vi "Dashboard Main (1).vi"() -> ()   [LabVIEW 2013]
uses:
  Shoot Profile.ctl
  Autonomous Setpoints.ctl
  Halo Drive.ctl
  Auto Speed Constants.ctl
  Auto Shift Settings.ctl
  Autonomous Center Line Setpoints.ctl
  UDP Dashboard Packet.ctl
  Shoot Location.ctl
  <vilib>/event_ctls.llb/eventvkey.ctl
  <vilib>/Utility/config.llb/Read Key (String).vi
  <vilib>/Utility/config.llb/Read Key (I32).vi
  <vilib>/Utility/config.llb/Write Key (String).vi
  <vilib>/Utility/config.llb/Write Key (I32).vi
  <vilib>/Utility/config.llb/NI_LVConfig.lvlib
  <vilib>/vision/NI_Vision_Development_Module.lvlib
panel:
  in  "Tab Control 2":enum32{"Page 1", "Page 2"}(tab)
  out "Shooter/Output/Vision Mode":bool
  in  "Shooter/Control/Manual RPM":bool=TRUE caption="Manual\n  RPM"
  out "Motor/Output/Elevator Motor":dbl caption="Motor Output"
  in  "Elevator/Manual Elevation":dbl=24.5 caption="Manual"
  in  "Elevator/Feed Angle":dbl=20.0 caption="Feed"
  in  "Elevator/Auto Enabled":bool=TRUE caption="Auto Elevator Enabled"
  out "Shooter/Output/Shooter Ready":bool caption="Shooter Ready"
  in  "Shooter/Pre Feeding":dbl=-0.15 caption="Feed Power"
  in  "Shooter/Main Feeding":dbl=-0.2 caption="Main Feed Pwr"
  in  "Shooter/Control/Manual Main RPM":dbl=4000.0 caption="Target RPM"
  in  "Shooter/Shooter Main":dbl=0.6 caption="Manual Pwr"
  in  "Shooter/Shooter Pre":dbl=0.5 caption="Manual Pwr"
  in  "Shooter/Manual Power":bool caption="Manual Pwr"
  in  "Shooter/Control/Manual Pre RPM":dbl=3500.0 caption="Manual"
  in  "Shooter/Control/RPM Max Percentage":dbl=1.02 caption="RPM Max Percentage"
  in  "Shooter/Control/RPM Min Percentage":dbl=0.99 caption="RPM Min Percentage"
  out "Shooter/Output/Flipper Output":bool caption="Load"
  out "Shooter/Output/RPM Ready":bool caption="RPM"
  out "Elevator/Output/Shoot Angle Ready":bool caption="Elevation"
  in  "Elevator/Manual Elevation Enabled":bool=TRUE caption="Manual\n Angle"
  in  "Elevator/Max Angle":dbl=55.0 caption="Max"
  in  "Elevator/Min Angle":dbl=18.0 caption="Min"
  in  "Elevator/Neutral Angle":dbl=25.8 caption="Neutral Angle"
  out "Shooter/Output/Azimuth Ready":bool caption="Azimuth"
  in  "Azimuth/Auto Enabled":bool caption="Enabled"
  out "Azimuth/Target Delta":dbl caption="Auto Azimuth Delta"
  in  "Azimuth/Tolerance":dbl=3.0 caption="Tolerance"
  out "Azimuth/X Output":dbl caption="X Output"
  out "Elevator/Neutral Angle Ready":bool caption="Ready"
  out "Elevator/Finding Neutral Angle":bool caption="Seeking"
  in  "Elevator/Pyramid Angle":dbl=31.0 caption="Pyramid"
  in  "Elevator/Neutral Enabled":bool=TRUE caption="Neutral\nEnabled"
  out "Shooter/Control/Vision Main RPM":dbl caption="RPM"
  out "Shooter/Control/Vision Pre RPM":dbl caption="Vision"
  out "Elevator/Vision Angle":dbl caption="Vision"
  in  "Shooter/Control/Pyramid Main RPM":dbl=4000.0 caption="Target RPM"
  in  "Shooter/Control/Pyramid Pre RPM":dbl=3500.0 caption="Pyramid"
  in  "Shooter/Control/Full Court Main RPM":dbl=4000.0 caption="Target RPM"
  in  "Shooter/Control/Full Court Pre RPM":dbl=3500.0 caption="Full Court"
  out "Shooter/Output/Pyramid Mode":bool
  out "Shooter/Output/Full Court Mode":bool
  in  "Elevator/Full Court Angle":dbl=25.8 caption="Full Court"
  out "Elevator/Output/Feed Mode":bool
  out "Elevator/Output/Vision Mode":bool
  out "Elevator/Output/Pyramid Mode":bool
  out "Elevator/Output/Full Court Mode":bool
  out "Shooter/Output/Feed Mode":bool
  out "Elevator/Target Angle":dbl caption="Setpoint"
  in  "Camera Settings":T1={"Frate Rate"=30, "Compression"=30, "Size"=1} {"Frate Rate" scale=1.0..30.0; "Size" items=["640x480", "320x240", "160x120"]}
  in  "Dashboard Tab 2":enum32{"Drive", "Debug", "Controls"}(tab)
  out "Elevator Enabled":bool caption="Elevator"
  out "fps":dbl format="%#.1g"
  out "Mbps 2":bool
  in  "DB Camera Config":bool
  in  "Enable":bool=TRUE
  out "Mbps":dbl format="%#.1g"
  out "Camera Image":T2(plugin-control)
  in  "Elevator Angle Offset":dbl(slide)=-0.3 caption="Angle Offset" scale=-5.0..5.0
  out "Azmuth Enabled":bool caption="Azimuth"
  out "Shooter/Output/Shooter Ready 2":bool caption="Shooter Ready"
  out "Shooter/Output/Flipper Output 2":bool caption="Load"
  out "Shooter/Output/RPM Ready 2":bool caption="RPM"
  out "Elevator/Output/Shoot Angle Ready 2":bool caption="Elevation"
  out "Shooter/Output/Azimuth Ready 2":bool caption="Azimuth"
  out "Elevator/Output/Target Angle 2":dbl caption="Target"
  out "Elevator/Angle 2":dbl caption="Angle"
  out "Vision/Target Found":bool caption="Target\nFound"
  out "Shoot Distance":dbl
  out "Gyro Angle":dbl(knob) caption="Gyro" scale=0.0..360.0
  out "Drive Gear":dbl caption="Gear"
  out "Auto/Load Ramp Down":bool caption="Ramp Down"
  in  "Dashboard Tab":T3(tab)
  out "Encoder/Right Ticks":dbl caption="Right"
  out "Encoder/Left Ticks":dbl caption="Left"
  out "Encoder/Right Speed":dbl caption="Right"
  out "Encoder/Left Speed":dbl caption="Left"
  out "Auto/Shooter Mode":string="--------" caption="Shooter Mode"
  out "Drive/Gear":dbl caption="Gear"
  out "Encoder/Right Dist":dbl caption="Right"
  out "Encoder/Left Dist":dbl caption="Left"
  out "Encoder/Average Dist":dbl caption="Encoder Distance"
  out "Sensor/Disc Count":dbl caption="Discs" format="%#_1f"
  out "Sensor/Gyro/Angle":dbl(knob) caption="Gyro" scale=0.0..360.0
  out "Auto/Disc Mode":string="--------" caption="Disc Mode"
  out "Lift/Ratchet Locked":bool caption="Ratchet Locked"
  out "Shoot Active Vision":bool caption="Ratchet Locked"
  out "Shoot Active Pyramid":bool caption="Ratchet Locked"
  out "Shoot Active Full Court":bool caption="Ratchet Locked"
  out "Shoot Active Half Court":bool caption="Ratchet Locked"
  out "Shoot Active Back Corner":bool caption="Ratchet Locked"
  out "Shoot Active Front Corner":bool caption="Ratchet Locked"
  in  "Shoot Pyramid":T4={"Pre RPM"=2800.0, "Main RPM"=3300.0, "Angle"=28.0} caption="Pyramid"
  in  "Shoot Full Court":T4={"Pre RPM"=4500.0, "Main RPM"=4800.0, "Angle"=12.0} caption="Full Court"
  in  "Shoot Half Court":T4={"Pre RPM"=3600.0, "Main RPM"=4100.0, "Angle"=16.4} caption="Half Court"
  in  "Shoot Front Corner":T4={"Pre RPM"=3600.0, "Main RPM"=4100.0, "Angle"=19.900000000000002} caption="Front Corner"
  in  "Shoot Front":T4={"Pre RPM"=3600.0, "Main RPM"=4100.0, "Angle"=23.5} caption="Front"
  out "Sensor/Shooter Pot/Value":dbl caption="Pot Voltage"
  in  "Angle Equation x0":dbl=51.125
  in  "Angle Equation x1":dbl=-2.486
  in  "Angle Equation x2":dbl=0.0385 caption="Vision Angle Equation"
  in  "Manual Elevation Enabled":bool=TRUE
  in  "Manual Angle":dbl=16.4
  out "Vision Elevation":dbl caption="Vision Angle"
  in  "Feed Angle":dbl=20.0
  in  "Neutral Angle":dbl=16.4
  in  "Shoot Vision":T4={"Pre RPM"=3600.0, "Main RPM"=4100.0, "Angle"=16.4}
  in  "Shooter/Control/Manual Dist Enabled":bool caption="Manual Distance"
  in  "Shooter/Control/Manual Dist":dbl=12.0 caption="Manual Distance"
  out "Camera Distance 2":dbl caption="Camera Dist"
  out "Shoot Distance 2":dbl caption="Shoot Dist"
  out "Shooter/Control/Target Pre RPM":dbl caption="Setpoint"
  out "Shooter/Control/Target Main RPM":dbl caption="RPM"
  out "Shooter/Output/Pre RPM":dbl caption="Sensor"
  out "Shooter/Output/Pre":dbl caption="Output"
  out "Shooter/Output/Main":dbl caption="Motor\nOutput"
  out "Shooter/Output/Main RPM":dbl caption="RPM"
  out "Elevator/Angle 3":dbl caption="Angle"
  out "Elevator/Output/Target Angle 3":dbl caption="Target"
  out "Shoot Active Front":bool caption="Ratchet Locked"
  in  "Shoot Back Corner":T4={"Pre RPM"=3600.0, "Main RPM"=4100.0, "Angle"=13.300000000000006} caption="Back Corner"
  in  "Angle Tolerance":dbl=0.1
  in  "Unjam Servo Angle":dbl=60.0
  in  "Potentiometer Angle":cluster{"Pot M":dbl, "Pot B":dbl}={"Pot M"=42.09, "Pot B"=-65.397}
  out "Elevator/Output/Target Angle":dbl caption="Target"
  in  "Sensor/Shooter Pot/Value":dbl caption="Shooter Pot"
  out "Elevator/Angle":dbl caption="Angle"
  in  "Halo Drive":T5={"Gains"={"Quickturn_Sens_Low"=1.2, "Quickturn_Sens_High"=0.85, "Speedturn_Sens_Low"=1.5, "Speedturn_Sens_High"=2.0}, "QuickTurn Const"=0.25, "Loading Throttle Limit"=0.5}
  in  "Toggle Ears Delay":dbl=-1.0
  in  "Left Roller Pwr":dbl=0.9
  in  "Right Roller Pwr":dbl=0.8
  in  "Toggle Ears Distance":dbl=2.0
  in  "Auto Shift":T6={"Enabled"=FALSE, "Upshift Speed"=6.0, "Downshift Speed"=2.0, "Upshift Throttle"=0.6000000000000001, "Turn Power Diff"=0.7, "Motor Limit"=100.0, "Encoder Limit"=1500.0}
  in  "Shooting Delays":T7={"Unjam On"=200.0, "Unjam Off"=200.0, "Flipper On"=200.0, "Flipper Off"=0.0, "Hopper Up"=300.0}
  in  "Auto Reverse Speed":dbl=0.5
  in  "Autonomous Setpoints":T8={"Shoot Angle 1"=14.8, "Initial Delay"=0.0, "Disc Count 1"=3.0, "Shoot Time 1"=8000.0, "Distance 1"=6.5, "Two Disc Distance 1"=4.0, "Distance 2"=12.5, "Two Disc Distance 2"=6.0, "Distance 3"=-11.8, "Two Disc Distance 3"=0.0, "Shoot Angle 3"=22.5, "Disc Count 3"=5.0, "Shoot Time 3"=15000.0, "Distance 4"=0.0, "Two Disc Distance 4"=0.0, "Low Gear"=TRUE, "Shoot 1 Post Delay"=250.0}
  in  "Auto Speed Constants":T9={"Slowing Distance"=0.5, "High Speed"=0.8999999999999999, "Rampup Time"=500.0, "Low Speed"=0.5, "High Speed (Reverse)"=0.8999999999999999}
  in  "Auto Stop Throttle":dbl
  in  "Auto Stop Duration (ms)":dbl
  in  "Auto-Center Line":T10={"Arc Turn x-axis"=0.0, "Arc Turn y-axis"=0.8999999999999999, "Arc Turn Distance"=-11.0, "Distance 1"=11.0, "Two Disc Distance 1"=0.0, "Distance 2"=-2.0, "Two Disc Distance 2"=0.0, "Spin Angle"=-70.0, "Spin Angle tolerance"=5.0, "Spin y-axis"=0.0, "Spin Distance"=0.0, "Center Line Enabled"=FALSE, "Distance 3"=11.999999999999998, "Two Disc Distance 3"=0.0, "Spin Angle 2"=85.0, "Spin Angle tolerance 2"=15.0, "Spin y-axis 2"=0.0, "Spin Distance 2"=0.0, "Shoot Angle 1"=14.6, "Disc Count 1"=3.0, "Shoot Time 1"=8000.0, "Shoot Angle 3"=18.4, "Disc Count 3"=5.0, "Shoot Time 3"=15000.0, "Low Gear"=TRUE}
  in  "Slider":dbl(slide) scale=0.0..100.0 scale format="%#_3g"
  in  "On/Off":bool caption="Solenoid"
  in  "Test Name":u16(ring) items=["Select the test to run...", "Example Test", "-------------------------------", "List of tests is built in robot code.", "Replace with your own automated tests."]
  in  "Test Tree":string(tree)
  in  "Motor":cluster{"Value":dbl, "Enable":bool} {"Value" scale=-1.0..1.0 scale format="%#_3g"}
  out "Progress":T11 {"Test Progress" scale=0.0..100.0}
  in  "Rev/Fwd":cluster{"Forward":bool, "Reverse":bool}
  in  "Ring":u16(ring) items=["Auto", "Fixed indoor", "Fixed outdoor 1", "Fixed outdoor 2", "Fixed fluorescent 1", "Fixed fluorescent 2", "Hold current"]
  in  "Listbox":i32(listbox)
  out "Tree":string(tree)
  out "UDP packet length":i32
  in  "Auton Distance output range\nCenter Line":cluster{"output high":dbl, "output low":dbl}={"output high"=1.0, "output low"=-1.0}
  in  "Auton Distance PID gains\nHigh Gear":T12={"proportional gain (Kc)"=0.26, "integral time (Ti, min)"=0.018000000000000002, "derivative time (Td, min)"=0.0}
  in  "Elevator PID Gains":T12={"proportional gain (Kc)"=0.2, "integral time (Ti, min)"=0.0, "derivative time (Td, min)"=0.002}
  in  "Elevator PID Output Range":cluster{"output high":dbl, "output low":dbl}={"output high"=1.0, "output low"=-1.0}
  in  "Auton Steer PID gains":T12={"proportional gain (Kc)"=0.4, "integral time (Ti, min)"=0.0, "derivative time (Td, min)"=0.002}
  in  "Auton Steer output range":cluster{"output high":dbl, "output low":dbl}={"output high"=0.5, "output low"=-0.5}
  in  "Auton Spin output range":cluster{"output high":dbl, "output low":dbl}={"output high"=1.0, "output low"=-1.0}
  in  "Auton Spin PID gains":T12={"proportional gain (Kc)"=0.4, "integral time (Ti, min)"=0.0, "derivative time (Td, min)"=0.0}
  in  "Auton Distance PID gains\nLow Gear":T12={"proportional gain (Kc)"=0.9999999999999999, "integral time (Ti, min)"=0.007, "derivative time (Td, min)"=0.0}
  in  "Auton Distance output range":cluster{"output high":dbl, "output low":dbl}={"output high"=0.93, "output low"=-0.93}
  in  "Auton Distance Threshold":dbl=0.5
  in  "Auton Velocity Cutoff":dbl=2.0
  in  "Mask":bool
  out "Image Display":T2(plugin-control)
  in  "View":bool
  in  "Tab Control":enum32{"Variables", "Calibration"}(tab)
  out "Target Info":T13(array[cluster])
  in  "Particle Count Limit":i32=8
  in  "Area Size Limit %":dbl=0.5
  in  "Score Limits":T14={"Rect Coverage"=60.0, "X Edge Strength"=40.0, "Y Edge Strength"=60.0, "Center"=75.0, "Outer"=75.0}
  in  "Camera Type":enum16{"206", "1011"}(ring)=enum."1011"
  out "Center Position":cluster{"X":dbl, "Y":dbl}
  out "Vision Distance (ft)":dbl caption="Distance (ft)"
  out "Center":bool
  out "Position X":dbl
  in  "Default Distance (ft)":dbl=14.0
  in  "Position to\nGyro constant":dbl=21.75
  in  "Azimuth Offset":dbl
  out "Azimuth/Target Delta 2":dbl caption="Auto Azimuth Delta"
  out "Azimuth/X Output 2":dbl caption="X Output"
  in  "Image Filter Values":T15={"Hue"=105, "Saturation"=255, "Luminance"=235, "Margins"={"Hue"=80, "Val"=80, "Sat"=0}} {"Margins"."Sat" scale=0.0..80.0; "Margins"."Val" scale=0.0..80.0; "Margins"."Hue" scale=0.0..80.0; "Hue" scale=0.0..255.0}
  out "Image Filter Ranges":T16
  out "Battery Value":dbl(slide) scale=0.0..14.0 scale format="%#_2e"
  out "Battery":sgl(graph)
  out "JS1 Z":dbl(slide) scale=-1.0..1.0 scale format="%#_2e"
  out "JS2 Z":dbl(slide) scale=-1.0..1.0 scale format="%#_2e"
  out "Joystick 1":cluster{"X":dbl, "Y":dbl}[](graph)
  out "Joystick 2":cluster{"X":dbl, "Y":dbl}[](graph)
  out "JS Buttons 1":T17
  out "JS Buttons 2":T17
  out "MotorSlide4":dbl(slide) scale=-1.0..1.0 scale format="%#_2e"
  out "MotorSlide3":dbl(slide) scale=-1.0..1.0 scale format="%#_2e"
  out "MotorSlide2":dbl(slide) scale=-1.0..1.0 scale format="%#_2e"
  in  "MotorName3":string="Front Left"
  in  "MotorName4":string="Front Right"
  in  "MotorName1":string="Rear Left"
  in  "MotorName2":string="Rear Right"
  out "MotorChart4":dbl(graph)
  out "MotorChart3":dbl(graph)
  out "MotorChart2":dbl(graph)
  out "MotorSlide1":dbl(slide) scale=-1.0..1.0 scale format="%#_2e"
  out "MotorChart1":dbl(graph)
  out "Robot IP":string
  out "Mode":T18(ring)=enum."Auto Disabled"
  out "Camera IP":string
  in  "Viewer":T19(tab)
  out "Image Error Message":string="Timeout in Camera Communications"
  out "Buttons 1":cluster{"1":bool, "2":bool, "3":bool}
  out "Kinect 1":cluster{"X":dbl, "Y":dbl, "Z":dbl} {"X" scale=1.0..-1.0; "Y" scale=1.0..-1.0; "Z" scale=1.0..-1.0}
  out "Buttons 2":cluster{"1":bool, "2":bool, "3":bool}
  out "Kinect 2":cluster{"X":dbl, "Y":dbl, "Z":dbl} {"X" scale=1.0..-1.0; "Y" scale=1.0..-1.0; "Z" scale=1.0..-1.0}
  out "Version":string
  out "Skeleton Picture":picture
  out "Players":i8
  # "Pre"
  # "Main"
  # "Neutral"
  # "Vision: 3500, 4000\nPyramid: 2800, 3200  39.1\nFull Court: 4300, 4800 18"
  # "Shooter"
  # "Elevator"
  # "Distance"
  # "Ticks"
  # "Speed"
  # "RPM"
  # "NOTE: used as\nBack angle"
  # "Pre RPM"
  # "Main RPM"
  # "Angle"
  # "Dpad UP"
  # "Elevator UP"
  # "Elevator DOWN"
  # "Dpad LEFT"
  # "Dpad RIGHT"
  # "[DISABLED]"
  # "Elevator"
  # "Whiteboard:                               y = -2.6332x + 68.073\nTesting 2.23.13                           y = 0.2002x2 - 7.6337x + 101.11\nTesting 2.24.13                           y = 0.2086x2 - 7.5585x + 94.621\nField Test (Orch room) 3.2.13  y = 0.0733x2 - 3.2492x + 59.29\nField Test (Orch room) 3.3.13  y = 0.0782x2 - 3.7527x + 65.268\nLonestar Thursday 3.7.13         y = 0.0872x2 - 3.5994x + 63.288 \nLonestar Friday 3.8.13               y = 0.178x2 - 6.8038x + 91.639\nPrePeachtree 3.11.13                 y = -0.0522x2 + 0.9287x + 27.34 \nPeachtree Thurs 3.14.13           y = -0.0766x2 + 0.7339x + 30.218\nPeachtree Thurs 3.14.13 PM    y = 0.0385x2 - 2.486x + 51.125"
  # "Dpad DOWN"
  # "x^2"
  # "x"
  # "Start angle: 28"
  # "Duration to move Lift Piston up\nat beginning of teleop (-1 to disable)"
  # "Quickturn - LOW throttle"
  # "Speedturn - HIGH throttle"
  # "Volts -> Degrees\ny = Mx + B"
  # "throttle value where Speedturn activates"
  # "Max throttle value when ramp is down"
  # "2 Corner:\nDistance 1 = 18\nDistance 2 = 0\nSpin 2 = 105\nDistance 3 = 10"
  # "Distance before stopping,\nswitch to low speed"
  # "Time to get to full speed (ms)"
  # "7.13.13\nP=0.6\nI =0.006\nD=0"
  # "2.23.13\nP=0.068\nI =0.8\nD=0.008\nTolerance=3deg"
  # "Original values:\np=0.3, range [-1, 1]"
  # "Original values:\n1.2, 1\n1.5, 1.7"
  # "Driver  [USB 1]"
  # "Manipulator [USB 2]"
  # "Drive & Motors"
  # "Simple Shoot: [2] (uses back pyramid angle)\nAdvanced Shoot:\n     Back of Pyramid:  [D-Pad Down] + [2]\n     Front of Pyramid: [D-Pad Up] + [2]\n     Front Corner: [11 Up] + [2]\n     Back Corner: [11 Down] + [2]\n     Half Court: [D-Pad Left] + [2]\n     Full Court:  [D-Pad Right] + [2]\nNOTE: [2] activates flipper (other button\nwarms up shooter & angle)\n\nLeft Roller -    [5] Forward; [7] Backward\nRight Roller - [6] Forward; [8] Backward\n\nFront Feeding - [3]\n\nManual Flipper - [9]\nManual Hopper - [1]\nManual Unjam - [12 Down]\nManual Elevator - [10] + [11 Up/Down]\n^(disables auto elevator, push [11] to re-enable)\nEnable Auto Elevator - [Push 11]\n\nVision Enabled - [4]*  (disabled by default)\n*toggle button"
  # "Drive:\n     Throttle - [11 Up/Down]\n     Steering - [12 Left/Right]\n     Gear Shift - [5]*\n     (starts in High gear)\n\n10pt Lift Piston - [7]* or [2]*\n\nAuto Load - [6]\nLoad Ramp Down - [8]\n\n*toggle button"
  # "Note: Most commonly used controls are listed first"
  # "Robot IP:"
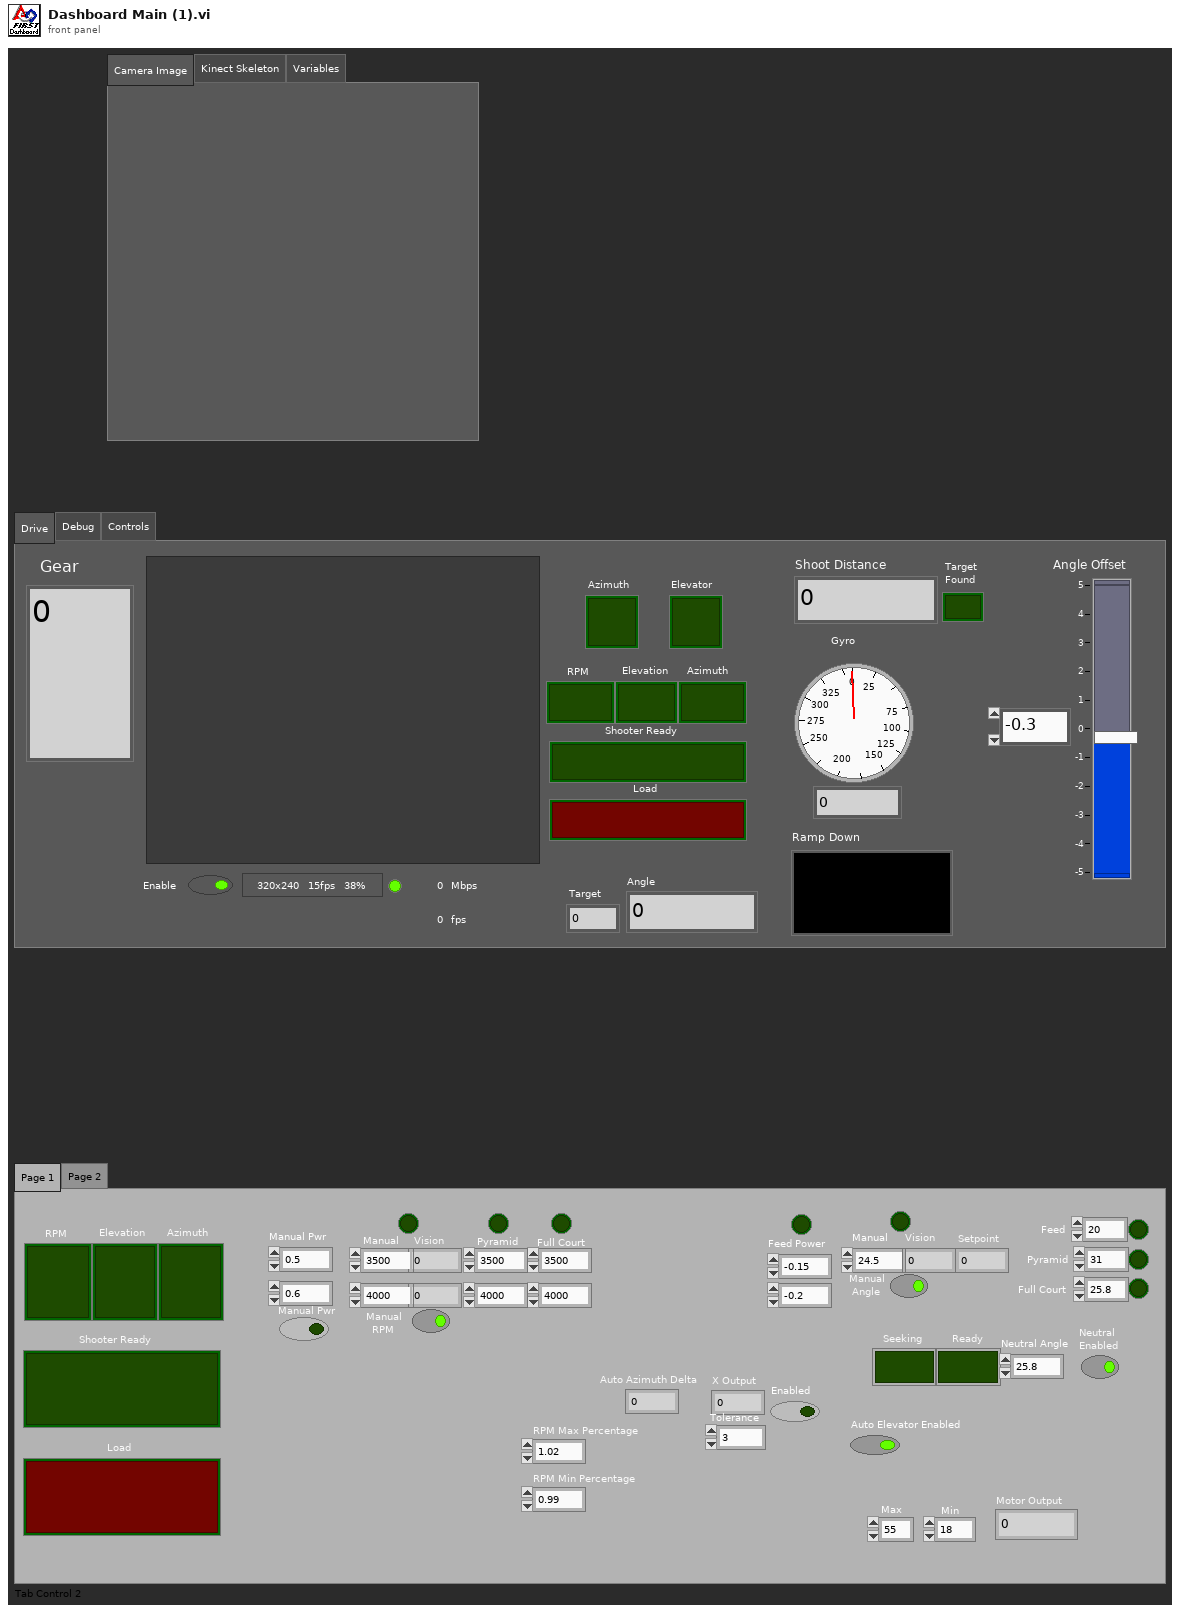
[diagram p1: front panel]
types:
  T1 = cluster{"Frate Rate":i32, "Compression":i32, "Size":u16}
  T2 = typedef "IMAQ Image.ctl" = refnum<image>
  T3 = enum32{"Operation", "Shooter", "Auto", "Autonomous", "Test", "Variables", "PID", "Vision"}
  T4 = typedef "Shoot Profile.ctl" = cluster{"Pre RPM":dbl, "Main RPM":dbl, "Angle":dbl}
  T5 = typedef "Halo Drive.ctl" = cluster{"Gains":cluster{"Quickturn_Sens_Low":dbl, "Quickturn_Sens_High":dbl, "Speedturn_Sens_Low":dbl, "Speedturn_Sens_High":dbl}, "QuickTurn Const":dbl, "Loading Throttle Limit":dbl}
  T6 = typedef "Auto Shift Settings.ctl" = cluster{"Enabled":bool, "Upshift Speed":dbl, "Downshift Speed":dbl, "Upshift Throttle":dbl, "Turn Power Diff":dbl, "Motor Limit":dbl, "Encoder Limit":dbl}
  T7 = cluster{"Unjam On":dbl, "Unjam Off":dbl, "Flipper On":dbl, "Flipper Off":dbl, "Hopper Up":dbl}
  T8 = typedef "Autonomous Setpoints.ctl" = cluster{"Shoot Angle 1":dbl, "Initial Delay":dbl, "Disc Count 1":dbl, "Shoot Time 1":dbl, "Distance 1":dbl, "Two Disc Distance 1":dbl, "Distance 2":dbl, "Two Disc Distance 2":dbl, "Distance 3":dbl, "Two Disc Distance 3":dbl, "Shoot Angle 3":dbl, "Disc Count 3":dbl, "Shoot Time 3":dbl, "Distance 4":dbl, "Two Disc Distance 4":dbl, "Low Gear":bool, "Shoot 1 Post Delay":dbl}
  T9 = typedef "Auto Speed Constants.ctl" = cluster{"Slowing Distance":dbl, "High Speed":dbl, "Rampup Time":dbl, "Low Speed":dbl, "High Speed (Reverse)":dbl}
  T10 = typedef "Autonomous Center Line Setpoints.ctl" = cluster{"Arc Turn x-axis":dbl, "Arc Turn y-axis":dbl, "Arc Turn Distance":dbl, "Distance 1":dbl, "Two Disc Distance 1":dbl, "Distance 2":dbl, "Two Disc Distance 2":dbl, "Spin Angle":dbl, "Spin Angle tolerance":dbl, "Spin y-axis":dbl, "Spin Distance":dbl, "Center Line Enabled":bool, "Distance 3":dbl, "Two Disc Distance 3":dbl, "Spin Angle 2":dbl, "Spin Angle tolerance 2":dbl, "Spin y-axis 2":dbl, "Spin Distance 2":dbl, "Shoot Angle 1":dbl, "Disc Count 1":dbl, "Shoot Time 1":dbl, "Shoot Angle 3":dbl, "Disc Count 3":dbl, "Shoot Time 3":dbl, "Low Gear":bool}
  T11 = cluster{"Test Progress":u8, "Test Progress Text":string}
  T12 = cluster{"proportional gain (Kc)":dbl, "integral time (Ti, min)":dbl, "derivative time (Td, min)":dbl}
  T13 = cluster{"Center Position":cluster{"X":dbl, "Y":dbl}, "Distance (ft)":dbl, "Center":bool}[]
  T14 = cluster{"Rect Coverage":dbl, "X Edge Strength":dbl, "Y Edge Strength":dbl, "Center":dbl, "Outer":dbl}
  T15 = cluster{"Hue":i32, "Saturation":i32, "Luminance":i32, "Margins":cluster{"Hue":i32, "Val":i32, "Sat":i32}}
  T16 = cluster{"Hue":cluster{i32, i32}, "Sat":cluster{i32, i32}, "Lum":cluster{i32, i32}}
  T17 = cluster{bool, bool, bool, bool, bool, bool, bool, bool, bool, bool, bool, bool}
  T18 = enum8{"Tele-Op Disabled", "Tele-Op Enabled", "Auto Disabled", "Auto Enabled", "Test Disabled", "Test Enabled", ""}
  T19 = enum32{"Camera Image", "Kinect Skeleton", "Variables"}
  T20 = typedef "UDP Dashboard Packet.ctl" = cluster{"Feed Angle":dbl, "Neutral Angle":dbl, "Autonomous Setpoints":T8, "Auto Shift":T6, "Elevator Angle Offset":dbl, "Potentiometer Angle":cluster{"Pot M":dbl, "Pot B":dbl}, "Shoot Setpoints":cluster{"Vision":T4, "Back Corner":T4, "Front":T4, "Front Corner":T4, "Half Court":T4, "Full Court":T4, "Pyramid":T4}, "Halo Drive":T5, "Auto Speed Constants":T9, "Shooting Delays":cluster{"Unjam On":dbl, "Unjam Off":dbl, "Flipper On":dbl, "Flipper Off":dbl, "Hopper Up":dbl}, "Left Roller Pwr":dbl, "Right Roller Pwr":dbl, "Elevator PID Gains":cluster{"proportional gain (Kc)":dbl, "integral time (Ti, min)":dbl, "derivative time (Td, min)":dbl}, "Elevator PID Output Range":cluster{"output high":dbl, "output low":dbl}, "Elevator Angle Tolerance":dbl, "Toggle Ears Delay":dbl, "Toggle Ears Distance":dbl, "Unjam Servo Angle":dbl, "Auton Steer PID gains":cluster{"proportional gain (Kc)":dbl, "integral time (Ti, min)":dbl, "derivative time (Td, min)":dbl}, "Auton Steer output range":cluster{"output high":dbl, "output low":dbl}, "Auto Reverse Speed":dbl, "Auto Stop Throttle":dbl, "Auto Stop Duration":dbl, "Spin output range":cluster{"output high":dbl, "output low":dbl}, "Spin PID gains":cluster{"proportional gain (Kc)":dbl, "integral time (Ti, min)":dbl, "derivative time (Td, min)":dbl}, "Auto-Center Line":T10, "Auton Distance PID gains Low Gear":cluster{"proportional gain (Kc)":dbl, "integral time (Ti, min)":dbl, "derivative time (Td, min)":dbl}, "Auton Distance output range":cluster{"output high":dbl, "output low":dbl}, "Auton Distance Threshold":dbl, "Auton Velocity Cutoff":dbl, "Auton Distance output range Center Line":cluster{"output high":dbl, "output low":dbl}, "Auton Distance PID gains High Gear":cluster{"proportional gain (Kc)":dbl, "integral time (Ti, min)":dbl, "derivative time (Td, min)":dbl}}
  T21 = typedef "Image Type" = u32
  T22 = enum32{"Operation", "Test", "Checklist", "Shooter", "Elevator", "Motors", "Solenoids", "Auto"}
  T23 = enum32{"Operation", "Test", "Checklist", "Shooter", "Motors"}
  T24 = typedef "LVBoundsTypeDef.ctl" = cluster{"Width":u32, "Height":u32}
  T25 = typedef "SkeletonTrackState.ctl" = enum32{"NotTracked", "PositionOnly", "Tracked"}
  T26 = cluster{"TrackingState":u8[], "Position":cluster{"x":sgl, "y":sgl, "z":sgl}, cluster{"x":sgl, "y":sgl, "z":sgl, sgl}[], "TrackState":T25}
  T27 = cluster{cluster{"ScaledToPercentRange":dbl, "ScaledToPercentRange":dbl, "ScaledToPercentRange":dbl}, cluster{bool, bool, bool}}[]
  T28 = cluster{cluster{"ScaledToPercentRange":dbl, "ScaledToPercentRange":dbl, "ScaledToPercentRange":dbl}, cluster{bool, bool, bool}}
  T29 = cluster{"ScaledToPercentRange":dbl, "ScaledToPercentRange":dbl, "ScaledToPercentRange":dbl}
  T30 = typedef "LVRectTypeDef.ctl" = cluster{"Left":i16, "Top":i16, "Right":i16, "Bottom":i16}
  T31 = cluster{"Center Position":cluster{"X":dbl, "Y":dbl}, "Distance (ft)":dbl, "Center":bool}
  T32 = cluster{"Competition mode":bool, "Robot Link":bool, "Autonomous":bool, "Enabled":bool, "E-Stop":bool, "Simulated":bool, "TestMode":bool, "Docked Window":bool}
  T33 = cluster{"Boolean Array[0]":bool, "Boolean Array[1]":bool, "Boolean Array[2]":bool, "Boolean Array[3]":bool, "Boolean Array[4]":bool, "Boolean Array[5]":bool, "Boolean Array[6]":bool, "Boolean Array[7]":bool, "Boolean Array[8]":bool, "Boolean Array[9]":bool, "Boolean Array[10]":bool, "Boolean Array[11]":bool}
  T34 = typedef "NI_LVConfig.lvlib/Config Data RefNum.ctl" = refnum<k1>
  T35 = typedef "eventvkey.ctl" = enum16{"ASCII", "Enter", "Return", "Shift", "Ctrl", "Alt", "Cmd", "Opt", "Caps", "NumLock", "Clear", "Break", "Up", "Down", "Left", "Right", "Insert", "Delete", "Home", "End", "PageUp", "PageDown", "Escape", "Help", "Pause", "ScrollLock", "F1", "F2", "F3", "F4", "F5", "F6", "F7", "F8", "F9", "F10", "F11", "F12", "F13", "F14", "F15", "F16", "F17", "F18", "F19", "F20", "F21", "F22", "F23", "F24", "Play", "VolumeUp", "VolumeDown", "Mute", "Two Byte Char"}
  T36 = typedef "Shoot Location.ctl" = enum16{"Vision", "Front", "Front Corner", "Back Corner", "Half Court", "Full Court", "Pyramid"}
  T37 = cluster{"Vision":T4, "Back Corner":T4, "Front":T4, "Front Corner":T4, "Half Court":T4, "Full Court":T4, "Pyramid":T4}
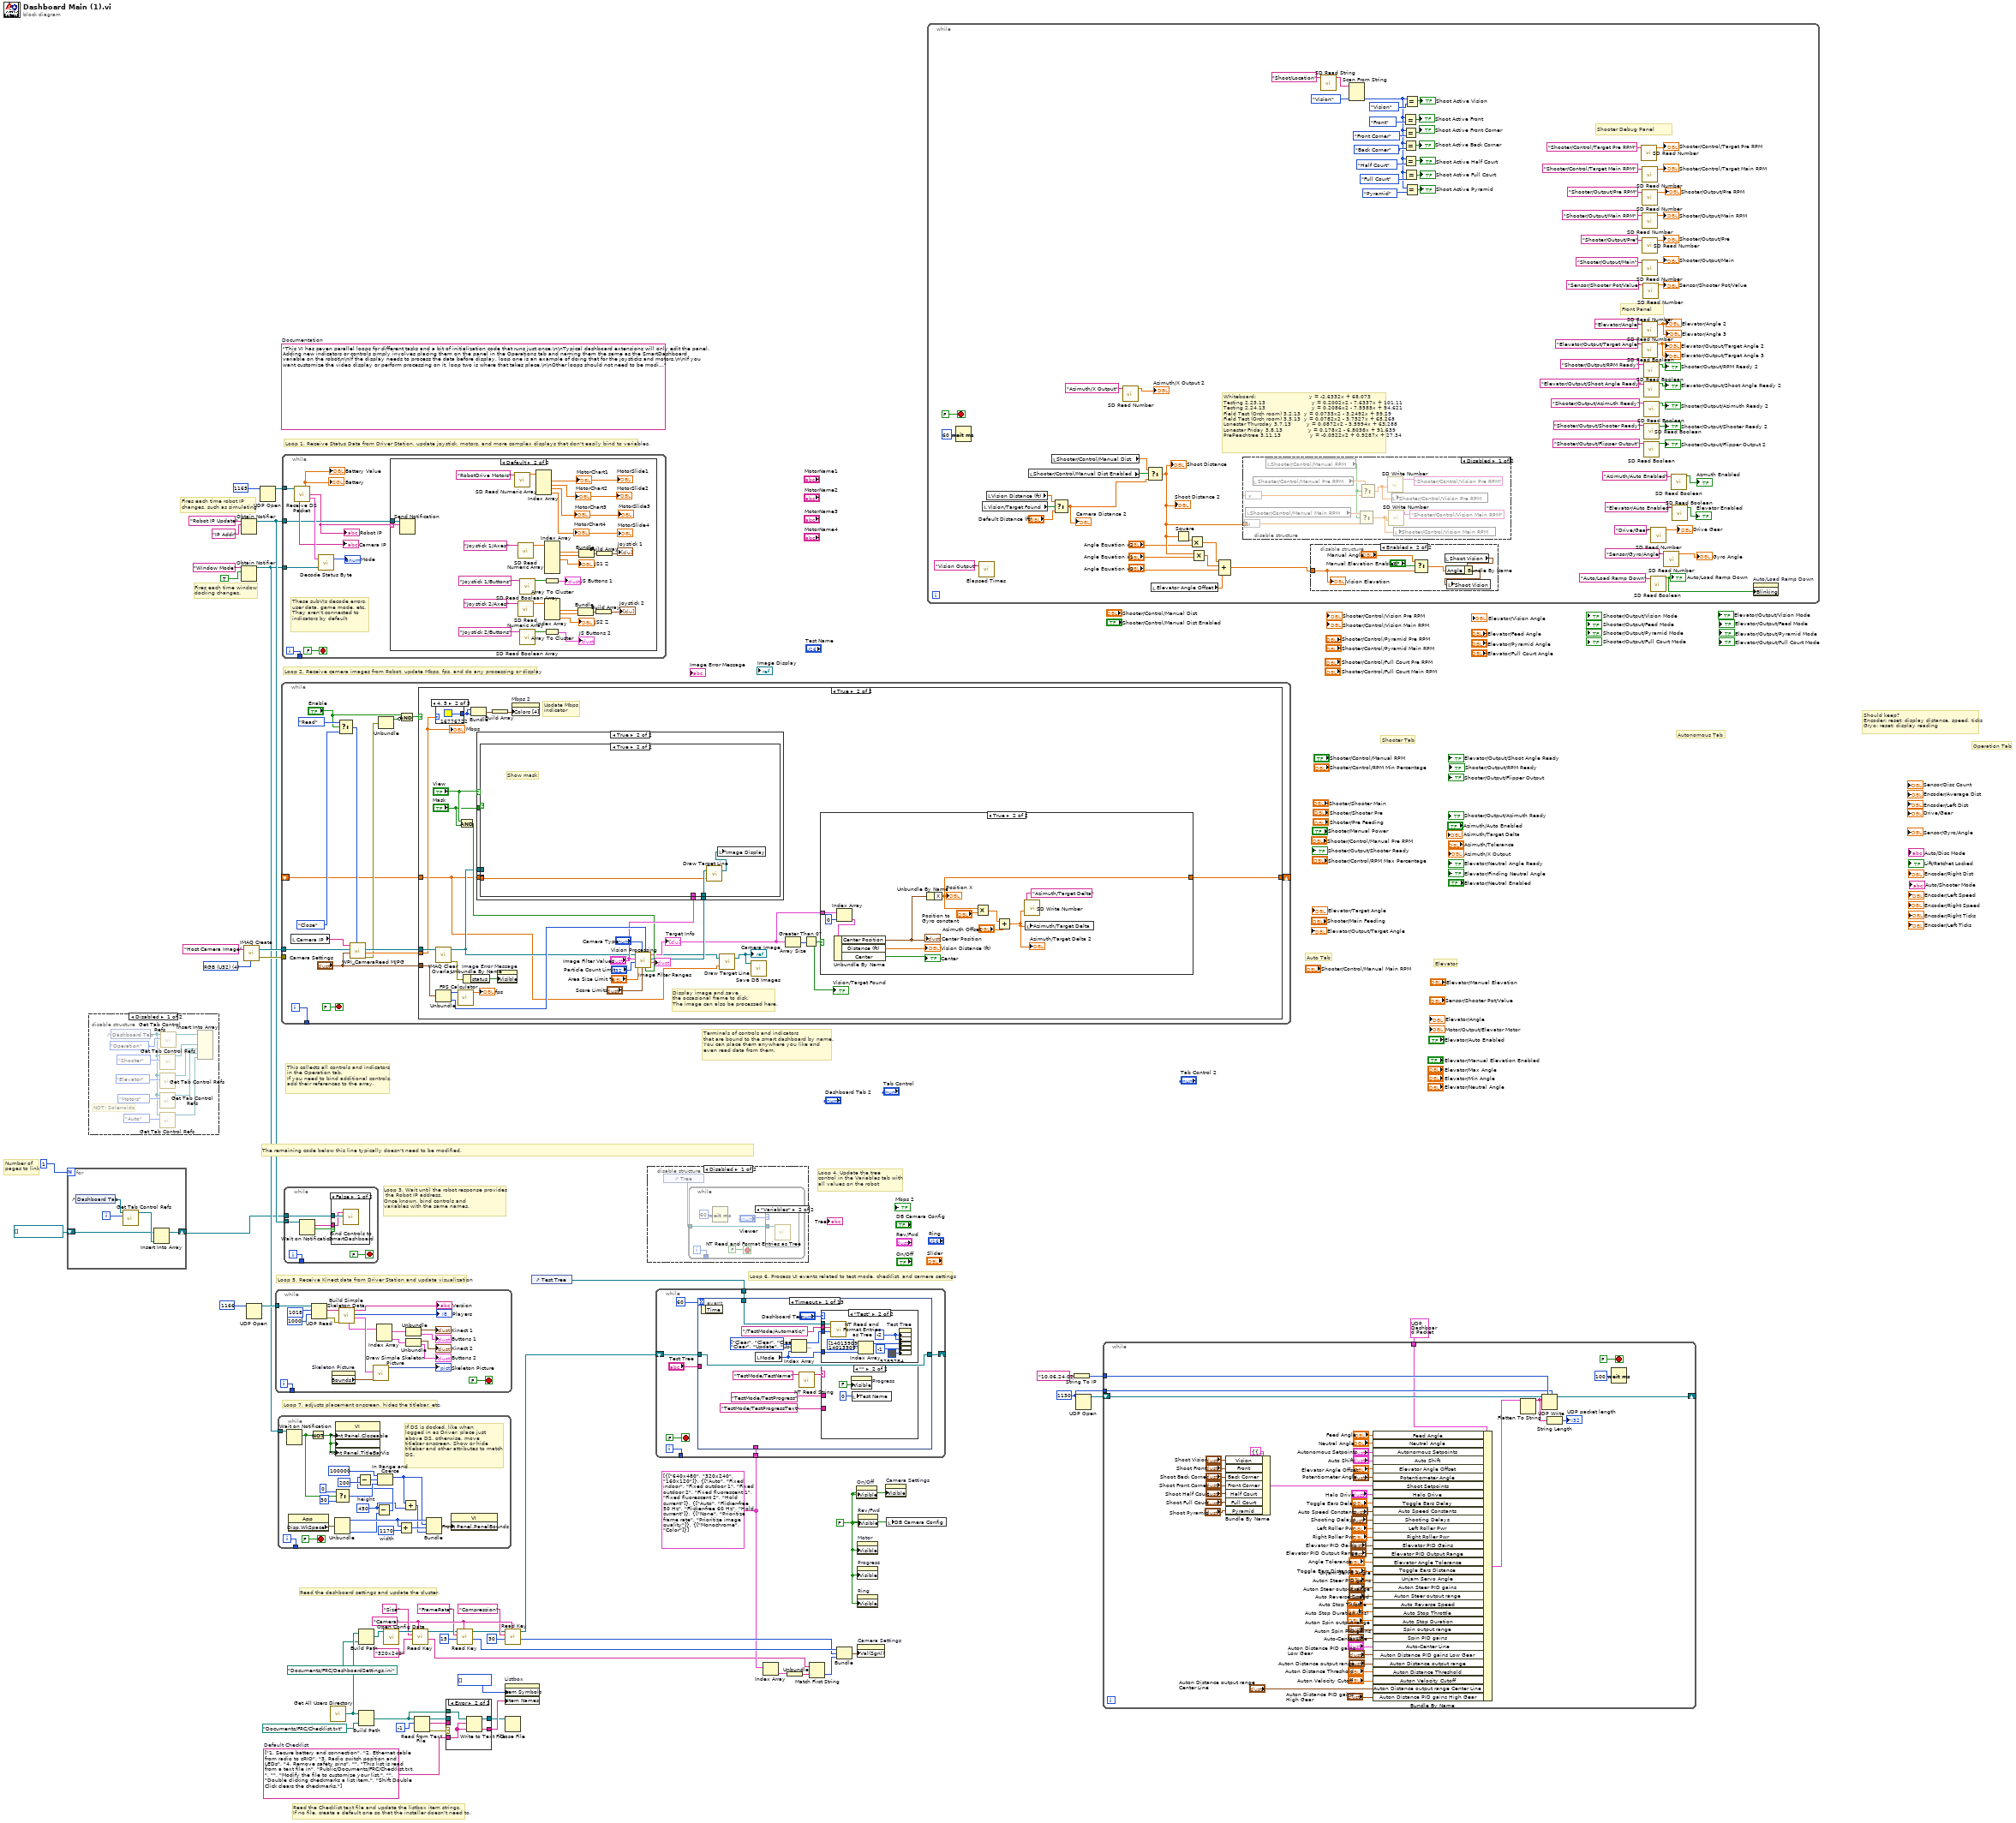
[diagram p0: block diagram]
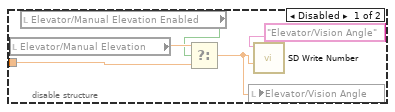
[diagram p2: hidden frame]
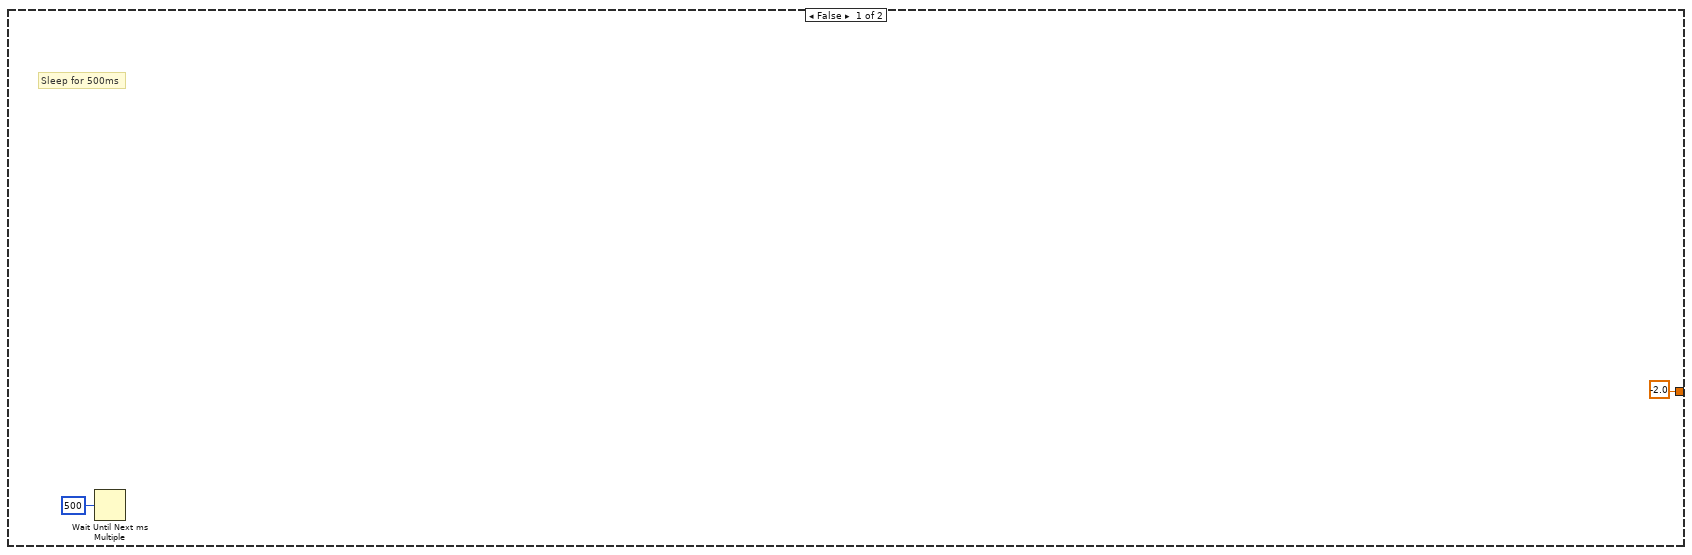
[diagram p8: hidden frame]
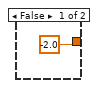
[diagram p9: hidden frame]
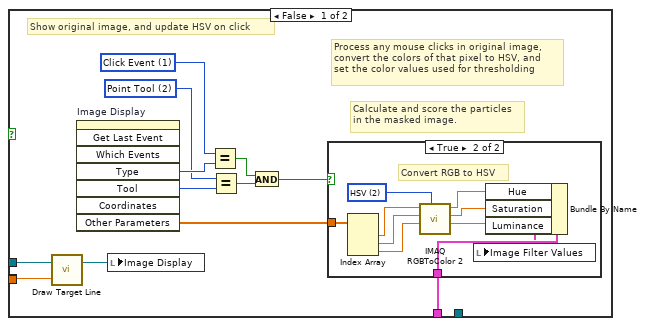
[diagram p11: hidden frame]
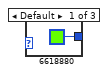
[diagram p13: hidden frame]
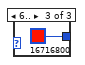
[diagram p14: hidden frame]
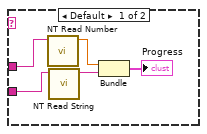
[diagram p17: hidden frame]
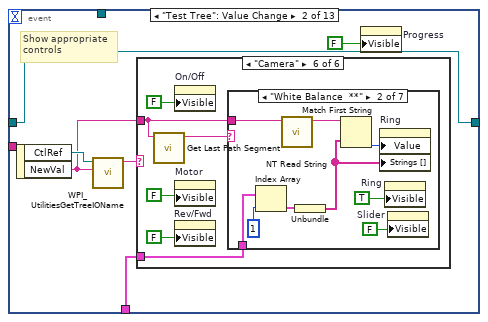
[diagram p18: hidden frame]
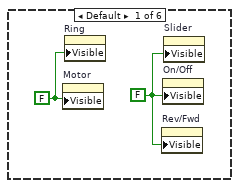
[diagram p19: hidden frame]
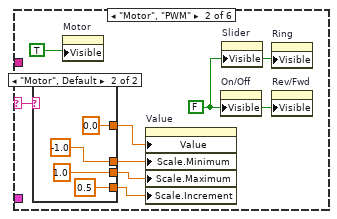
[diagram p20: hidden frame]
diagram:
  w2 = u16 1130 ("port")
  w28 = "Camera"
  w20 = cluster{string[]}[] [{["640x480", "320x240", "160x120"]}, {["Auto", "Fixed indoor", "Fixed outdoor 1", "Fixed outdoor 2", "Fixed fluorescent 1", "Fixed fluorescent 2", "Hold current"]}, {["Auto", "Flicker-free 50 Hz", "Flicker-free 60 Hz", "Hold current"]}, {["None", "Prioritize frame rate", "Prioritize image quality"]}, {["Monochrome", "Color"]}]
  w36 = string[] ["1. Secure battery and connection", "2. Ethernet cable from radio to cRIO", "3. Radio switch position and LEDs", "4. Remove safety pins", "", "This list is read from a text file in", "Public/Documents/FRC/Checklist.txt.", "", "Modify the file to customize your list.", "", "Double clicking checkmarks a list item.", "Shift Double Click clears the checkmarks."]  # Default Checklist
  w34 = FALSE ("Visible")
  (unwired) "This VI has seven parallel loops for different tasks and a bit of initialization code that runs just once.\n\nTypical dashboard extensions will only edit the panel. Adding new indicators or controls simply involves placing them on the panel in the Operations tab and naming them the same as the SmartDashboard variable on the robot\n\nIf the display needs to process the data before display, loop one is an example of doing that for the joysticks and motors.\n\nIf you want customize the video display or perform processing on it, loop two is where that takes place.\n\nOther loops should not need to be modified. They are pretty standard, and document the task they perform."  # Documentation
  w54 = T21 4 items=["Grayscale (U8)", "Grayscale (I16)", "Grayscale (SGL)", "Complex (CSG)", "RGB (U32)", "HSL (U32)", "RGB (U64)"] ("Image Type")
  # "Should keep?\nEncoder: reset; display distance, speed, ticks\nGryo: reset; display reading"
  # "Number of\npages to link"
  # "Autonomous Tab"
  # "Elevator"
  # "Auto Tab"
  # "Operation Tab"
  # "Shooter Tab"
  # "Fires each time robot IP\nchanges, such as simulating"
  # "Fires each time window\ndocking changes."
  # "Read the Checklist text file and update the listbox item strings.\nIf no file, create a default one so that the installer doesn't need to."
  # "This collects all controls and indicators\nin the Operation tab.\nIf you need to bind additional controls,\nadd their references to the array."
  # "The remaining code below this line typically doesn't need to be modified."
  # "Loop 6. Process UI events related to test mode, checklist, and camera settings"
  # "Read the dashboard settings and update the cluster."
  # "Terminals of controls and indicators\nthat are bound to the smart dashboard by name.\nYou can place them anywhere you like and\neven read data from them."
  # "Loop 4. Update the tree\ncontrol in the Variables tab with\nall values on the robot"
  # "Loop 3. Wait until the robot response provides\n the Robot IP address.\nOnce known, bind controls and\nvariables with the same names."
  # "Loop 5. Receive Kinect data from Driver Station and update visualization"
  # "Loop 7. adjusts placement onscreen, hides the titlebar, etc."
  # "Loop 1. Receive Status Data from Driver Station, update joystick, motors, and more complex displays that don't easily bind to variables."
  # "Loop 2. Receive camera images from Robot, update Mbps, fps, and do any processing or display"
  n1 = for {
    N: 1 -> [_]
    shift-right: [w58] -> w6
    shift-left: refnum<vi>[] [] -> [w57]
    i -> [w60]
    n2 = control-ref of="Dashboard Tab"() -> (w61:refnum<vi>)
    n3 = call <vilib>:"Get Tab Control Refs.vi"("Page Index"=w60, "TabControl in"=w61) -> ("ControlsOnPage"=w59:refnum<vi>[])  [unwired: 9 in]
    n4 = Insert Into Array(array=w57, new element=w59) -> (w58:refnum<vi>[])  [unwired: 1 in]
  }
  n5 = disable-structure shown="Disabled" {
    frame Disabled {
      # "NOT: Solenoids"
      n6 = control-ref of="Dashboard Tab"() -> (w62:refnum<vi>)
      n7 = call <vilib>:"Get Tab Control Refs.vi"("Page Index"=T22."Elevator" ("Dashboard Tab"), "TabControl in"=w62) -> ("ControlsOnPage"=w67:refnum<vi>[])  [unwired: 9 in]
      n8 = call <vilib>:"Get Tab Control Refs.vi"("Page Index"=T22."Motors" ("Dashboard Tab"), "TabControl in"=w62) -> ("ControlsOnPage"=w64:refnum<vi>[])  [unwired: 9 in]
      n9 = call <vilib>:"Get Tab Control Refs.vi"("Page Index"=T22."Auto" ("Dashboard Tab"), "TabControl in"=w62) -> ("ControlsOnPage"=w63:refnum<vi>[])  [unwired: 9 in]
      n10 = call <vilib>:"Get Tab Control Refs.vi"("Page Index"=T23."Shooter" ("Dashboard Tab"), "TabControl in"=w62) -> ("ControlsOnPage"=w71:refnum<vi>[])  [unwired: 9 in]
      n11 = call <vilib>:"Get Tab Control Refs.vi"("Page Index"=T23."Operation" ("Dashboard Tab"), "TabControl in"=w62) -> ("ControlsOnPage"=w70:refnum<vi>[])  [unwired: 9 in]
      n12 = Insert Into Array(array=w70, new element #1=w71, new element #2=w67, new element #3=w64, new element #4=w63) -> ()  [unwired: 1 in, 1 out]
    }
    frame Enabled {
    }
  }
  n13 = Obtain Notifier(name (unnamed)="Robot IP Update", notification data type="IP Addr" ("name (unnamed)")) -> (notifier out=w46:refnum<notifier>)  [unwired: 2 in, 2 out]
  n14 = Obtain Notifier(name (unnamed)="Window Mode", notification data type=TRUE) -> (notifier out=w40:refnum<notifier>)  [unwired: 2 in, 2 out]
  n15 = call "IMAQ Create"("Image Name"="Host Camera Image", "Image Type"=w54) -> ("New Image"=w52:T2, "error out"=w51:errorcluster)  [unwired: 2 in, 1 out]
  n16 = UDP Open(11:u16 1166 ("port")) -> (port=w49:refnum<k16>)  [unwired: 2 in, 4 out]
  n17 = UDP Open(11:u16 1165 ("port")) -> (port=w55:refnum<k16>)  [unwired: 2 in, 4 out]
  n18 = while {
    tunnel: w49 -> [w89]
    tunnel: [w74] -> _
    i -> [w74]
    stop <- FALSE stop-if-true
    n19 = UDP Read(connection ID=w89, max size (548)=1018 ("bytes to read"), timeout ms (25000)=1000) -> (data out=w83:string, error out=w73:errorcluster)  [unwired: 1 in, 3 out]
    n20 = property on="Skeleton Picture" class="Pict"() -> ("Bounds"=w85:T24)  [unwired: 2 in, 2 out]
    n21 = call "Build Simple Skeleton Data.vi"("error in (no error)"=w73, "data in"=w83) -> ("Skeleton Data"=w84:T26, "NumPlayers"=→"Players":i8, "Version String"=→"Version":string, "Simple Joystick Info"=w81:T27)  [unwired: 5 in, 1 out]
    n22 = call "Draw Simple Skeleton Picture.vi"("Bounds"=w85, "Simple Skeleton"=w84) -> ("new picture out"=→"Skeleton Picture":picture)  [unwired: 9 in]
    n23 = Index Array(array=w81) -> (element #1=w80:T28, element #2=w79:T28)  [unwired: 2 in]
    n24 = Unbundle(w80) -> (→"Kinect 1":T29, →"Buttons 1":cluster{bool, bool, bool})
    n25 = Unbundle(w79) -> (→"Kinect 2":T29, →"Buttons 2":cluster{bool, bool, bool})
  }
  n26 = while {
    tunnel: w40 -> [w111]
    tunnel: [w109] -> _
    i -> [w109]
    stop <- FALSE stop-if-true
    w103 = 1170  # width
    w92 = 450  # height
    # "If DS is docked, like when\nlogged in as Driver, place just\nabove DS, otherwise, move\ntitlebar onscreen. Show or hide\ntitlebar and other attributes to match\nDS."
    n27 = Wait on Notification(notifier=w111) -> (notification=w98:bool)  [unwired: 3 in, 3 out]
    n28 = property class="App"() -> ("Disp.WkSpace"=w107:T30)  [unwired: 2 in, 2 out]
    n29 = Not(x=w98) -> (.not. x?=w110:bool)
    n30 = Unbundle(w107) -> ("Left"=w105:i16, "Bottom"=w94:i16)  [unwired: 2 out]
    n31 = Select(t=0, s=w98, f=30) -> (s? t:f=w97:i32)
    n32 = property class="VI"("Front Panel.Closeable"=w110, "Front Panel.Minimizeable"=w110, "Front Panel.TitleBarVis"=w110) -> ()  [unwired: 2 in, 2 out]
    n33 = Subtract(x=w92, y=w94) -> (x-y=w93:i32)
    n34 = Subtract(x=w93, y=200) -> (x-y=w101:i32)
    n35 = In Range and Coerce(upper limit=100000, x=w101, lower limit=w97) -> (coerced(x)=w95:i32)  [unwired: 1 out]
    n36 = Add(x=w105, y=w103) -> (x+y=w106:i32)
    n37 = Add(x=w95, y=w92) -> (x+y=w104:i32)
    n38 = Bundle("Left"=w105, w95, w106, w104) -> (w108:cluster{"Left":i16, i32, i32, i32})  [unwired: 1 out]
    n39 = property class="VI"("Front Panel.PanelBounds"=w108) -> ()  [unwired: 2 in, 2 out]
  }
  n40 = while {
    tunnel: w52 -> [w124]
    tunnel: w51 -> [_]
    tunnel: [w127] -> _
    shift-right: [w114] -> _
    shift-left: _ -> [w113]
    i -> [w127]
    stop <- FALSE stop-if-true
    n41 = local read "Camera IP"() -> (w126:string)
    n42 = Select(t=enum16{"Read", "Reopen", "Close"}."Read" ("Operation"), s="Enable", f=enum16{"Read", "Reopen", "Close"}."Close" ("Operation")) -> (s? t:f=w119:enum16{"Read", "Reopen", "Close"})
    n43 = call <vilib>:"WPI_CameraRead MJPG.vi"("Operation"=w119, "Camera Settings"="Camera Settings", "Image"=w124, "address"=w126) -> ("error out"=w118:errorcluster, "Bandwidth (Mbps)"=w122:dbl, "Image Out"=w123:T2)  [unwired: 5 in]
    n44 = Unbundle(w118) -> ("status"=w116:bool)  [unwired: 2 out]
    n45 = Compound Arithmetic op=AND("Enable", invert w116) -> (w115:bool)
    n46 = case shown="True" w115 {
      tunnel: "Camera Settings" -> [_ w150]
      tunnel: w123 -> [_ w153]
      tunnel: w122 -> [_ w152]
      tunnel: [-2.0 ("X") w134] -> w114
      tunnel: w113 -> [_ w132]
      frame False {
        # "Sleep for 500ms"
        n47 = Wait Until Next ms Multiple(millisecond multiple=u32 500) -> ()  [unwired: 1 out]
      }
      frame True {
        # "Display image and save\nthe occasional frame to disk.\nThe image can also be processed here."
        # "Update Mbps\nindicator"
        n48 = call "IMAQ Clear Overlay"("Image"=w153) -> ("error out"=w157:errorcluster, "Image Out"=w133:T2)  [unwired: 2 in, 7 out]
        n49 = case shown="4, 5" w152 {
          tunnel: [u32 6618880 ("Color Box") u32 16776722 ("Color Box") u32 16716800 ("Color Box")] -> w154
          frame Default {
          }
          frame 4, 5 {
          }
          frame 6.. {
          }
        }
        n50 = Unbundle(w150) -> ("Frate Rate"=w149:i32, "Size"=w144:u16)  [unwired: 1 out]
        n51 = call "FPS Calculator.vi"("Average Count"=w149) -> ("fps"=→"fps":dbl)  [unwired: 10 in]
        n52 = And(x="View", y="Mask") -> (x .and. y?=w139:bool)
        n53 = Unbundle By Name(w157) -> ("status"=w158:bool)
        n54 = Bundle("Color Box"=w154, "Color Box"=w154) -> (w156:cluster{"Color Box":u32, "Color Box":u32})  [unwired: 1 out]
        n55 = Build Array(w156) -> (w155:cluster{"Color Box":u32, "Color Box":u32}[])
        n56 = property on="Image Error Message" class="Str"("Visible"=w158) -> ()  [unwired: 2 in, 2 out]
        n57 = property on="Mbps 2" class="Bool (strict)"("Colors [4]"=w155) -> ()  [unwired: 2 in, 2 out]
        n58 = call "Vision Processing.vi"("View Processed Image"=w139, "Image Size"=w144, "Score Limits"="Score Limits", "Camera Type"="Camera Type", "Area Size Limit %"="Area Size Limit %", "Particle Count Limit"="Particle Count Limit", "Image Filter Values"="Image Filter Values", "Image In"=w133) -> ("Image Filter Ranges"=→"Image Filter Ranges":T16, "Processed Image"=w142:T2, "Target Info"=w137:T13)  [unwired: 1 in]
        "Target Info" <- w137
        n59 = case shown="True" "View" {
          tunnel: w133 -> [_ w176]
          tunnel: "Image Filter Values" -> [_ w175]
          tunnel: "Mask" -> [_ w174]
          tunnel: w142 -> [_ w173]
          tunnel: w132 -> [_ w172]
          frame False {
            # "View disabled"
          }
          frame True {
            n60 = case shown="True" w174 {
              tunnel: w176 -> [w179 _]
              tunnel: w175 -> [w186 _]
              tunnel: w172 -> [w177 _]
              tunnel: w173 -> [_ w201]
              tunnel: w172 -> [_ w200]
              frame False {
                w180 = 2 items=["None", "Selection Tool", "Point Tool", "Line Tool", "Rectangle Tool", "Oval Tool", "Polygon Tool", "ClosedFreehandTool", "Annulus Tool", "Rotated Rectangle Tool", "Zoom Tool", "Pan Tool", "Polyline Tool", "Freehand Tool"] ("Tool")
                w181 = 1 items=["No Event"=0, "Click Event"=1, "Draw Event"=2, "Size Event"=4, "Scroll Event"=5, "Double Click Event"=8] ("Type")
                # "Show original image, and update HSV on click"
                # "Process any mouse clicks in original image,\nconvert the colors of that pixel to HSV, and\nset the color values used for thresholding"
                # "Calculate and score the particles\nin the masked image."
                n61 = call "Draw Target Line.vi"("X"=w177, "Image In"=w179) -> ("Image Out"=w178:T2)  [unwired: 1 in]
                n62 = invoke on="Image Display" class="ImageControl" method="Get Last Event"() -> ("Type"=w182:i32, "Tool"=w185:i32, "Other Parameters"=w187:sgl[])  [unwired: 8 in, 5 out]
                n63 = local write "Image Display"(w178) -> ()
                n64 = Equal?(x=w181, y=w182) -> (x = y?=w183:bool)
                n65 = Equal?(x=w180, y=w185) -> (x = y?=w184:bool)
                n66 = And(x=w183, y=w184) -> (x .and. y?=w188:bool)
                n67 = case shown="True" w188 {
                  tunnel: w187 -> [_ w198]
                  tunnel: w186 -> [_ w193]
                  frame False {
                  }
                  frame True {
                    w197 = u16 2 items=["RGB", "HSL", "HSV", "HSI", "CIE L*a*b*", "CIE XYZ"] ("Color Mode")
                    # "Convert RGB to HSV"
                    n68 = Index Array(array=w198) -> (element #1=w196:sgl, element #2=w195:sgl, element #3=w194:sgl)  [unwired: 3 in]
                    n69 = call "IMAQ RGBToColor 2"("Color Mode"=w197, "Blue value"=w194, "Green value"=w195, "Red value"=w196) -> ("Blue or Luma or Val or Inten or Z or b*value"=w189:dbl, "Green or Sat or Y or a* value"=w190:dbl, "Red or Hue or X or L* value"=w191:dbl)  [unwired: 4 in, 1 out]
                    n70 = Bundle By Name(cluster=w193, "Hue"=w191, "Saturation"=w190, "Luminance"=w189) -> (w192:T15)
                    n71 = local write "Image Filter Values"(w192) -> ()
                  }
                }
              }
              frame True {
                # "Show mask"
                n72 = call "Draw Target Line.vi"("X"=w200, "Image In"=w201) -> ("Image Out"=w199:T2)  [unwired: 1 in]
                n73 = local write "Image Display"(w199) -> ()
              }
            }
          }
        }
        n74 = call "Draw Target Line.vi"("X"=w132, "Image In"=w133) -> ("Image Out"=w131:T2)  [unwired: 1 in]
        "Camera Image" <- w131
        n75 = call "Save DB Images.vi"("Image"=w131) -> ()  [unwired: 2 in, 1 out]
        n76 = Array Size(array=w137) -> (size(s)=w138:i32)
        n77 = Greater Than 0?(x=w138) -> (x > 0?=w136:bool)
        "Vision/Target Found" <- w136
        n78 = case shown="True" w136 {
          tunnel: w137 -> [_ w171]
          tunnel: [-2.0 ("X") w163] -> w134
          frame False {
          }
          frame True {
            n79 = Index Array(array=w171, index=0) -> (element=w169:T31)
            n80 = Unbundle By Name(w169) -> ("Center Position"=w166:cluster{"X":dbl, "Y":dbl}, "Distance (ft)"=→"Vision Distance (ft)":dbl, "Center"=→"Center":bool)
            "Center Position" <- w166
            n81 = Unbundle By Name(w166) -> ("X"=w163:dbl)
            "Position X" <- w163
            n82 = Multiply(x=w163, y="Position to\nGyro constant") -> (x*y=w161:dbl)
            n83 = Add(x=w161, y="Azimuth Offset") -> (x+y=w160:dbl)
            "Azimuth/Target Delta 2" <- w160
            n84 = call <vilib>:"SD Write Number.vi"("Numeric"=w160, "Name"="Azimuth/Target Delta") -> ()  [unwired: 8 in, 2 out]
            n85 = local write "Azimuth/Target Delta"(w160) -> ()
          }
        }
        "Mbps" <- w152
      }
    }
  }
  n86 = while {
    tunnel: w55 -> [w212]
    tunnel: w46 -> [w206]
    tunnel: w40 -> [w210]
    tunnel: [w207] -> _
    i -> [w207]
    stop <- FALSE stop-if-true
    # "These subVIs decode errors, user data, game mode, etc.\nThey aren't connected to indicators by default"
    n87 = call "Receive DS Packet.vi"("Recv Socket"=w212) -> ("Battery"=→"Battery" →"Battery Value":sgl, "Robot IP Address"=w205:string, "Status"=w213:T32, "Camera IP Address"=→"Camera IP":string)  [unwired: 1 in, 10 out]
    "Robot IP" <- w205
    n88 = call "Decode Status Byte.vi"("Window Mode Notifier"=w210, "Status"=w213) -> ("Mode"=→"Mode":T18)  [unwired: 1 out]
    n89 = case shown="Default" w205 {
      selector: w205 -> [_ w215]
      tunnel: w206 -> [_ w216]
      frame "0.0.0.0" {
        # "Robot not responding, don't poll the variables"
      }
      frame Default {
        n90 = Send Notification(notification=w215, notifier=w216) -> ()  [unwired: 1 in, 2 out]
        n91 = call <vilib>:"SD Read Numeric Array.vi"("Name"="RobotDrive Motors") -> ("Numeric Array"=w239:dbl[])  [unwired: 8 in, 2 out]
        n92 = call <vilib>:"SD Read Numeric Array.vi"("Name"="Joystick 1/Axes") -> ("Numeric Array"=w232:dbl[])  [unwired: 8 in, 2 out]
        n93 = call <vilib>:"SD Read Numeric Array.vi"("Name"="Joystick 2/Axes") -> ("Numeric Array"=w226:dbl[])  [unwired: 8 in, 2 out]
        n94 = call <vilib>:"SD Read Boolean Array.vi"("Name"="Joystick 1/Buttons") -> ("Boolean Array"=w234:bool[])  [unwired: 8 in, 2 out]
        n95 = call <vilib>:"SD Read Boolean Array.vi"("Name"="Joystick 2/Buttons") -> ("Boolean Array"=w225:bool[])  [unwired: 8 in, 2 out]
        n96 = Index Array(array=w239) -> (element #1=→"MotorChart1" →"MotorSlide1":dbl, element #2=→"MotorSlide2" →"MotorChart2":dbl, element #3=→"MotorChart3" →"MotorSlide3":dbl, element #4=→"MotorChart4" →"MotorSlide4":dbl)  [unwired: 4 in]
        n97 = Array To Cluster(array=w234) -> (cluster=→"JS Buttons 1":T33)
        n98 = Array To Cluster(array=w225) -> (cluster=→"JS Buttons 2":T33)
        n99 = Index Array(array=w232) -> (element #1=w229:dbl, element #2=w230:dbl, element #3=→"JS1 Z":dbl)  [unwired: 6 in, 3 out]
        n100 = Index Array(array=w226) -> (element #1=w221:dbl, element #2=w220:dbl, element #3=→"JS2 Z":dbl)  [unwired: 3 in]
        n101 = Bundle("Numeric"=w221, "Numeric"=w220) -> (w222:cluster{"Numeric":dbl, "Numeric":dbl})  [unwired: 1 in]
        n102 = Bundle("Numeric"=w229, "Numeric"=w230) -> (w228:cluster{"Numeric":dbl, "Numeric":dbl})  [unwired: 1 in]
        n103 = Build Array(w222) -> (→"Joystick 2":cluster{"Numeric":dbl, "Numeric":dbl}[])
        n104 = Build Array(w228) -> (→"Joystick 1":cluster{"Numeric":dbl, "Numeric":dbl}[])
      }
    }
  }
  n105 = while {
    tunnel: w6 -> [w248]
    tunnel: w46 -> [w245]
    tunnel: [w243] -> _
    i -> [w243]
    stop <- FALSE stop-if-true
    n106 = Wait on Notification(notifier=w245) -> (notification=w244:string, timed out?=w246:bool)  [unwired: 3 in, 2 out]
    n107 = case shown="False" w246 {
      tunnel: w248 -> [w250 _]
      tunnel: w244 -> [w249 _]
      frame False {
        n108 = call <vilib>:"Bind Controls to SmartDashboard.vi"("Bound Control Refs"=w250, "Server IP Address"=w249) -> ()  [unwired: 10 in]
      }
      frame True {
      }
    }
  }
  n109 = call "Get All Users Directory.vi"() -> ("All User Path"=w33:path)
  n110 = Build Path(base path=w33, name or relative path=path "Documents/FRC/DashboardSettings.ini") -> (appended path=w32:path)
  n111 = Build Path(base path=w33, name or relative path=path "Documents/FRC/Checklist.txt") -> (appended path=w37:path)
  n112 = call <vilib>:"Open Config Data.vi"("configuration file path"=w32) -> ("refnum"=w31:T34)  [unwired: 8 in, 2 out]
  n113 = call-poly <vilib>:"Read Key.vi"("section"=w28, "default value"="320x240", "key"="Size", "refnum"=w31) -> ("value"=w18:string, "refnum out"=w13:T34)  [unwired: 2 in, 4 out]
  n114 = Read from Text File(file (use dialog)=w37, count=-1 ("timeout ms (25000)")) -> (refnum out=w15:refnum<file>, text=w38:string[], error out=w39:errorcluster)  [unwired: 2 in, 1 out]
  n115 = case shown="Error" w39 {
    tunnel: w38 -> [w252 _]
    tunnel: [w252 w254] -> w35
    tunnel: w36 -> [_ w254]
    tunnel: w37 -> [_ w255]
    tunnel: [w251 w253] -> w14
    tunnel: w15 -> [w251 _]
    frame No Error {
    }
    frame Error {
      n116 = Write to Text File(file (use dialog)=w255, text=w254) -> (refnum out=w253:refnum<file>)  [unwired: 2 in, 2 out]
    }
  }
  n117 = call-poly <vilib>:"Read Key.vi"("section"=w28, "default value"=15, "key"="FrameRate", "refnum"=w13) -> ("value"=w23:i32, "refnum out"=w12:T34)  [unwired: 1 in, 5 out]
  n118 = property on="Listbox" class="LstBox (strict)"("Item Symbols"=i32[] [], "Item Names"=w35) -> ()  [unwired: 2 in, 2 out]
  n119 = Close File(refnum=w14) -> ()  [unwired: 1 in, 2 out]
  n120 = call-poly <vilib>:"Read Key.vi"("section"=w28, "default value"=30, "key"="Compression", "refnum"=w12) -> ("value"=w22:i32, "refnum out"=w10:T34)  [unwired: 1 in, 5 out]
  n121 = control-ref of="Test Tree"() -> (w9:refnum<vi>)
  n122 = disable-structure shown="Disabled" {
    frame Disabled {
      n123 = control-ref of="Tree"() -> (w256:refnum<vi>)
      n124 = while {
        tunnel: [w258] -> _
        tunnel: w256 -> [w257]
        i -> [w258]
        stop <- FALSE stop-if-true
        n125 = Wait (ms)(milliseconds to wait=u32 60) -> ()  [unwired: 1 out]
        n126 = case shown="\"Variables\"" "Viewer" {
          tunnel: w257 -> [_ w262]
          frame Default {
          }
          frame "Variables" {
            n127 = call <vilib>:"NT Read and Format Entries as Tree.vi"("Tree Refnum"=w262) -> ()  [unwired: 9 in, 2 out]
          }
        }
      }
    }
    frame Enabled {
    }
  }
  n128 = while {
    tunnel: w20 -> [w267]
    shift-right: [w266] -> _
    shift-left: w10 -> [w265]
    tunnel: [w264] -> _
    tunnel: w9 -> [w263]
    i -> [w264]
    stop <- FALSE stop-if-true
    n129 = event shown="[0] Timeout" {
      selector: _ -> [_ _ _ _ _ _ _ _ _ _ _ _ _]
      dyn-events: _ -> [_ _ _ _ _ _ _ _ _ _ _ _ _]
      timeout: u32 60 ("milliseconds to wait") -> [_ _ _ _ _ _ _ _ _ _ _ _ _]
      tunnel: w263 -> [w277 _ _ _ _ _ _ _ _ _ _ _ _]
      tunnel: "Test Tree" -> [_ _ _ _ _ _ _ _ w471 w479 w481 w485 w493]
      tunnel: w267 -> [_ w299 _ _ _ _ w435 w465 _ _ _ _ _]
      tunnel: [w271 w298 _ w401 w409 w421 w434 w458 w470 w477 w480 w484 w492] -> w266
      tunnel: w265 -> [w271 w298 _ w401 w409 w421 w433 w458 w470 w477 w480 w484 w492]
      event Timeout {
        w276 = enum16{"Update", "Clear"}[] [enum."Clear", enum."Clear", enum."Clear", enum."Clear", enum."Update", enum."Update", enum."Clear"] items=["Update", "Clear"]
        n130 = event-data() -> ()  [unwired: 1 in, 1 out]
        n131 = local read "Mode"() -> (w274:T18)
        n132 = Index Array(array=w276, index=w274) -> (element=w275:enum16{"Update", "Clear"})
        n133 = call <vilib>:"NT Read String.vi"("Name"="TestMode/TestName") -> ("String"=w280:string)  [unwired: 9 in, 1 out]
        n134 = case shown="\"Test\"" "Dashboard Tab" {
          tunnel: w277 -> [_ w290]
          tunnel: "/TestMode/Automatic/" ("Name Pattern") -> [_ w289]
          tunnel: w275 -> [_ w288]
          tunnel: w274 -> [_ w286]
          frame "Operation", Default {
          }
          frame "Test" {
            w285 = -2 ("Active Item:Row Number")
            n135 = call <vilib>:"NT Read and Format Entries as Tree.vi"("Operation"=w288, "Name Pattern"=w289, "Tree Refnum"=w290) -> ()  [unwired: 7 in, 2 out]
            n136 = Index Array(array=u32[] [14013909, 14013909, 14013909, 14013909, 14013909, 16777215, 14013909], index=w286) -> (element=w284:u32)
            n137 = property on="Test Tree" class="Tree (strict)"("Active Item Row Number"=w285, "ActiveColNum"=w285, "CellBG"=w284, "Active Item Row Number"=-1 ("Active Item:Row Number"), "CellBG"=u32 5789784 ("Color Box")) -> ()  [unwired: 2 in, 2 out]
          }
        }
        n138 = case shown="\"\"" w280 {
          tunnel: "TestMode/TestProgress" ("Name") -> [w292 _]
          tunnel: "TestMode/TestProgressText" ("Name") -> [w291 _]
          frame Default {
            n139 = call <vilib>:"NT Read Number.vi"("Name"=w292) -> ("Numeric"=w293:dbl)  [unwired: 9 in, 1 out]
            n140 = call <vilib>:"NT Read String.vi"("Name"=w291) -> ("String"=w294:string)  [unwired: 9 in, 1 out]
            n141 = Bundle("Numeric"=w293, "String"=w294) -> (→"Progress":cluster{"Numeric":dbl, "String":string})  [unwired: 1 in]
          }
          frame "" {
            n142 = property on="Progress" class="Clust (strict)"("Visible"=FALSE) -> ()  [unwired: 2 in, 2 out]
            n143 = local write "Test Name"(u16 0) -> ()
          }
        }
      }
      event "Test Tree": Value Change {
        # "Show appropriate\ncontrols"
        n144 = event-data() -> ("CtlRef"=w302:refnum<vi>, "NewVal"=w300:string)  [unwired: 1 in]
        n145 = call <vilib>:"WPI_UtilitiesGetTreeIOName.vi"("NewVal"=w300, "TreeControl in"=w302) -> ("I/O Name"=w303:string)  [unwired: 9 in]
        n146 = case shown="\"Camera\"" w303 {
          selector: w303 -> [_ w310 _ w328 w337 _]
          tunnel: w300 -> [_ _ w325 w327 _ w344]
          tunnel: w299 -> [_ _ _ _ _ w343]
          frame Default {
            w305 = FALSE ("Visible")
            w304 = FALSE ("Visible")
            n147 = property on="Motor" class="Clust (strict)"("Visible"=w304) -> ()  [unwired: 2 in, 2 out]
            n148 = property on="Ring" class="Ring (strict)"("Visible"=w304) -> ()  [unwired: 2 in, 2 out]
            n149 = property on="Rev/Fwd" class="Clust (strict)"("Visible"=w305) -> ()  [unwired: 2 in, 2 out]
            n150 = property on="On/Off" class="Bool (strict)"("Visible"=w305) -> ()  [unwired: 2 in, 2 out]
            n151 = property on="Slider" class="Slide (strict)"("Visible"=w305) -> ()  [unwired: 2 in, 2 out]
          }
          frame "Motor", "PWM" {
            w311 = FALSE ("Visible")
            n152 = case shown="\"Motor\", Default" w310 {
              tunnel: [1.0 ("Value") -1.0 ("Value")] -> w309
              tunnel: [255.0 ("Value") 1.0 ("Value")] -> w308
              tunnel: [128.0 ("Value") 0.0 ("Value")] -> w307
              tunnel: [64.0 ("Value") 0.5 ("Value")] -> w306
              frame "PWM" {
              }
              frame "Motor", Default {
              }
            }
            n153 = property on="Motor" class="Clust (strict)"("Visible"=TRUE) -> ()  [unwired: 2 in, 2 out]
            n154 = property on="Value" class="Slide (strict)"("Value"=w307, "Scale.Minimum"=w309, "Scale.Maximum"=w308, "Scale.Increment"=w306) -> ()  [unwired: 2 in, 2 out]
            n155 = property on="On/Off" class="Bool (strict)"("Visible"=w311) -> ()  [unwired: 2 in, 2 out]
            n156 = property on="Slider" class="Slide (strict)"("Visible"=w311) -> ()  [unwired: 2 in, 2 out]
            n157 = property on="Ring" class="Ring (strict)"("Visible"=w311) -> ()  [unwired: 2 in, 2 out]
            n158 = property on="Rev/Fwd" class="Clust (strict)"("Visible"=w311) -> ()  [unwired: 2 in, 2 out]
          }
          frame "Servo" {
            w323 = FALSE ("Visible")
            n159 = call <vilib>:"NT Read Number.vi"("Name"=w325) -> ("Numeric"=w324:dbl)  [unwired: 9 in, 1 out]
            n160 = property on="Slider" class="Slide (strict)"("Visible"=TRUE, "Scale.Maximum"=170.0 ("Scale.Range:Maximum")) -> ()  [unwired: 2 in, 2 out]
            n161 = local write "Slider"(w324) -> ()
            n162 = property on="Motor" class="Clust (strict)"("Visible"=w323) -> ()  [unwired: 2 in, 2 out]
            n163 = property on="Rev/Fwd" class="Clust (strict)"("Visible"=w323) -> ()  [unwired: 2 in, 2 out]
            n164 = property on="On/Off" class="Bool (strict)"("Visible"=w323) -> ()  [unwired: 2 in, 2 out]
            n165 = property on="Ring" class="Ring (strict)"("Visible"=w323) -> ()  [unwired: 2 in, 2 out]
          }
          frame "Relay", "Solenoid" {
            w326 = FALSE ("Visible")
            n166 = property on="Motor" class="Clust (strict)"("Visible"=w326) -> ()  [unwired: 2 in, 2 out]
            n167 = property on="Slider" class="Slide (strict)"("Visible"=w326) -> ()  [unwired: 2 in, 2 out]
            n168 = Search and Replace String(input string=w327, search string="/Value  **", replace string="/Direction") -> (result string=w333:string)  [unwired: 5 in, 3 out]
            n169 = property on="Ring" class="Ring (strict)"("Visible"=w326) -> ()  [unwired: 2 in, 2 out]
            n170 = call <vilib>:"NT Read String.vi"("Name"=w333) -> ("String"=w331:string)  [unwired: 9 in, 1 out]
            n171 = Equal?(x="Both directions", y=w331) -> (x = y?=w329:bool)
            n172 = Not(x=w329) -> (.not. x?=w330:bool)
            n173 = property on="Rev/Fwd" class="Clust (strict)"("Visible"=w329) -> ()  [unwired: 2 in, 2 out]
            n174 = property on="On/Off" class="Bool (strict)"("Visible"=w330, "Caption.Text"=w328) -> ()  [unwired: 2 in, 2 out]
          }
          frame "Compressor", "Digital Out" {
            w336 = FALSE ("Visible")
            # "Get direction and finish"
            n175 = property on="Motor" class="Clust (strict)"("Visible"=w336) -> ()  [unwired: 2 in, 2 out]
            n176 = property on="Slider" class="Slide (strict)"("Visible"=w336) -> ()  [unwired: 2 in, 2 out]
            n177 = property on="Ring" class="Ring (strict)"("Visible"=w336) -> ()  [unwired: 2 in, 2 out]
            n178 = property on="On/Off" class="Bool (strict)"("Visible"=TRUE, "Caption.Text"=w337) -> ()  [unwired: 2 in, 2 out]
            n179 = property on="Rev/Fwd" class="Clust (strict)"("Visible"=FALSE) -> ()  [unwired: 2 in, 2 out]
          }
          frame "Camera" {
            n180 = call <vilib>:"Get Last Path Segment.vi"("String in"=w344) -> ("String out"=w345:string)  [unwired: 10 in]
            n181 = property on="On/Off" class="Bool (strict)"("Visible"=FALSE) -> ()  [unwired: 2 in, 2 out]
            n182 = property on="Motor" class="Clust (strict)"("Visible"=FALSE) -> ()  [unwired: 2 in, 2 out]
            n183 = property on="Rev/Fwd" class="Clust (strict)"("Visible"=FALSE) -> ()  [unwired: 2 in, 2 out]
            n184 = case shown="\"White Balance  **\"" w345 {
              tunnel: w344 -> [w351 w360 w369 w378 w387 _ w393]
              tunnel: w343 -> [w349 w357 w366 w375 w384 _ _]
              frame "Size  **" {
                n185 = Index Array(array=w349) -> (element=w348:cluster{string[]})  [unwired: 1 in]
                n186 = call <vilib>:"NT Read String.vi"("Name"=w351) -> ("String"=w350:string)  [unwired: 9 in, 1 out]
                n187 = Unbundle(w348) -> (w346:string[])
                n188 = Match First String(2:w346, 3:w350) -> (0:w347:i32)  [unwired: 1 out]
                n189 = property on="Ring" class="Ring (strict)"("Value"=w347, "Strings []"=w346) -> ()  [unwired: 2 in, 2 out]
                n190 = property on="Ring" class="Ring (strict)"("Visible"=TRUE) -> ()  [unwired: 2 in, 2 out]
                n191 = property on="Slider" class="Slide (strict)"("Visible"=FALSE) -> ()  [unwired: 2 in, 2 out]
              }
              frame "White Balance  **" {
                n192 = Index Array(array=w357, index=1) -> (element=w358:cluster{string[]})
                n193 = call <vilib>:"NT Read String.vi"("Name"=w360) -> ("String"=w359:string)  [unwired: 9 in, 1 out]
                n194 = Unbundle(w358) -> (w355:string[])
                n195 = Match First String(2:w355, 3:w359) -> (0:w354:i32)  [unwired: 1 out]
                n196 = property on="Ring" class="Ring (strict)"("Value"=w354, "Strings []"=w355) -> ()  [unwired: 2 in, 2 out]
                n197 = property on="Ring" class="Ring (strict)"("Visible"=TRUE) -> ()  [unwired: 2 in, 2 out]
                n198 = property on="Slider" class="Slide (strict)"("Visible"=FALSE) -> ()  [unwired: 2 in, 2 out]
              }
              frame "Exposure  **" {
                n199 = Index Array(array=w366, index=2) -> (element=w367:cluster{string[]})
                n200 = call <vilib>:"NT Read String.vi"("Name"=w369) -> ("String"=w368:string)  [unwired: 9 in, 1 out]
                n201 = Unbundle(w367) -> (w363:string[])
                n202 = Match First String(2:w363, 3:w368) -> (0:w364:i32)  [unwired: 1 out]
                n203 = property on="Ring" class="Ring (strict)"("Value"=w364, "Strings []"=w363) -> ()  [unwired: 2 in, 2 out]
                n204 = property on="Ring" class="Ring (strict)"("Visible"=TRUE) -> ()  [unwired: 2 in, 2 out]
                n205 = property on="Slider" class="Slide (strict)"("Visible"=FALSE) -> ()  [unwired: 2 in, 2 out]
              }
              frame "Exposure Priority  **" {
                n206 = Index Array(array=w375, index=3) -> (element=w376:cluster{string[]})
                n207 = call <vilib>:"NT Read String.vi"("Name"=w378) -> ("String"=w377:string)  [unwired: 9 in, 1 out]
                n208 = Unbundle(w376) -> (w372:string[])
                n209 = Match First String(2:w372, 3:w377) -> (0:w373:i32)  [unwired: 1 out]
                n210 = property on="Ring" class="Ring (strict)"("Value"=w373, "Strings []"=w372) -> ()  [unwired: 2 in, 2 out]
                n211 = property on="Ring" class="Ring (strict)"("Visible"=TRUE) -> ()  [unwired: 2 in, 2 out]
                n212 = property on="Slider" class="Slide (strict)"("Visible"=FALSE) -> ()  [unwired: 2 in, 2 out]
              }
              frame "Color Enable  **" {
                n213 = Index Array(array=w384, index=4) -> (element=w385:cluster{string[]})
                n214 = call <vilib>:"NT Read String.vi"("Name"=w387) -> ("String"=w386:string)  [unwired: 9 in, 1 out]
                n215 = Unbundle(w385) -> (w381:string[])
                n216 = Match First String(2:w381, 3:w386) -> (0:w382:i32)  [unwired: 1 out]
                n217 = property on="Ring" class="Ring (strict)"("Value"=w382, "Strings []"=w381) -> ()  [unwired: 2 in, 2 out]
                n218 = property on="Ring" class="Ring (strict)"("Visible"=TRUE) -> ()  [unwired: 2 in, 2 out]
                n219 = property on="Slider" class="Slide (strict)"("Visible"=FALSE) -> ()  [unwired: 2 in, 2 out]
              }
              frame Default {
                n220 = property on="Ring" class="Ring (strict)"("Visible"=FALSE) -> ()  [unwired: 2 in, 2 out]
                n221 = property on="Slider" class="Slide (strict)"("Visible"=FALSE) -> ()  [unwired: 2 in, 2 out]
              }
              frame "Brightness  **", "Color Level  **", "Compression  **", "FPS  **", "Sharpness  **" {
                n222 = call <vilib>:"NT Read Number.vi"("Name"=w393) -> ("Numeric"=w392:dbl)  [unwired: 9 in, 1 out]
                n223 = local write "Slider"(w392) -> ()
                n224 = property on="Slider" class="Slide (strict)"("Visible"=TRUE, "Scale.Maximum"=100.0 ("Scale.Range:Maximum")) -> ()  [unwired: 2 in, 2 out]
                n225 = property on="Ring" class="Ring (strict)"("Visible"=FALSE) -> ()  [unwired: 2 in, 2 out]
              }
            }
          }
        }
        n226 = property on="Progress" class="Clust (strict)"("Visible"=FALSE) -> ()  [unwired: 2 in, 2 out]
      }
      event "Test Name": Mouse Enter {
        # "Populate the ring with the list of tests"
        n227 = event-data() -> ()  [unwired: 1 in, 1 out]
        n228 = call <vilib>:"NT Read String Array.vi"("Name"="TestMode/TestList") -> ("String Array"=w400:string[])  [unwired: 9 in, 1 out]
        n229 = Build Array (concatenate)("Select the test to run...", w400) -> (w399:string[])
        n230 = property on="Test Name" class="Ring (strict)"("Strings []"=w399) -> ()  [unwired: 2 in, 2 out]
      }
      event "Test Name": Value Change {
        w402 = FALSE ("Visible")
        # "Tell the robot the test name to run"
        n231 = event-data() -> ("NewVal"=w406:u16)  [unwired: 1 in]
        n232 = property on="Test Name" class="Ring (strict)"() -> ("Strings []"=w407:string[])  [unwired: 2 in, 2 out]
        n233 = local write "Progress"(T11 {"Test Progress"=0, "Test Progress Text"=""} ("Progress")) -> ()
        n234 = Index Array(array=w407, index=w406) -> (element=w405:string)
        n235 = call <vilib>:"NT Write String.vi"("String"=w405, "Name"="TestMode/TestName") -> ()  [unwired: 9 in, 1 out]
        n236 = property on="Progress" class="Clust (strict)"("Visible"=TRUE) -> ()  [unwired: 2 in, 2 out]
        n237 = property on="Motor" class="Clust (strict)"("Visible"=w402) -> ()  [unwired: 2 in, 2 out]
        n238 = property on="Slider" class="Slide (strict)"("Visible"=w402) -> ()  [unwired: 2 in, 2 out]
        n239 = property on="On/Off" class="Bool (strict)"("Visible"=w402) -> ()  [unwired: 2 in, 2 out]
        n240 = property on="Rev/Fwd" class="Clust (strict)"("Visible"=w402) -> ()  [unwired: 2 in, 2 out]
        n241 = property on="Ring" class="Ring (strict)"("Visible"=w402) -> ()  [unwired: 2 in, 2 out]
      }
      event "Listbox": Double Click {
        n242 = event-data() -> ("PlatMods.Shift"=w410:bool, "Row"=w412:i32)  [unwired: 1 in]
        n243 = case shown="False" w410 {
          tunnel: w412 -> [w416 _]
          tunnel: 1 -> [w415 _]
          frame False {
            n244 = property on="Listbox" class="LstBox (strict)"() -> ("Item Symbols"=w414:i32[])  [unwired: 2 in, 2 out]
            n245 = Replace Array Subset(array=w414, new element=w415, index=w416) -> (w413:i32[])
            n246 = property on="Listbox" class="LstBox (strict)"("Item Symbols"=w413) -> ()  [unwired: 2 in, 2 out]
          }
          frame True {
            w417 = 0 ("Top Row")
            n247 = property on="Listbox" class="LstBox (strict)"() -> ("Number of Rows"=w419:u32)  [unwired: 2 in, 2 out]
            n248 = Initialize Array(0, w419) -> (w418:i32[])
            n249 = property on="Listbox" class="LstBox (strict)"("Top Row"=w417, "Value"=w417, "Item Symbols"=w418) -> ()  [unwired: 2 in, 2 out]
          }
        }
      }
      event "Listbox": Key Down {
        n250 = event-data() -> ("VKey"=w423:T35)  [unwired: 1 in]
        n251 = case shown="\"Left\", \"Right\"" w423 {
          selector: w423 -> [w428 _]
          tunnel: eventvkey."Left" ("VKey") -> [w426 _]
          frame "Left", "Right" {
            n252 = Equal?(x=w426, y=w428) -> (x = y?=w427:bool)
            n253 = Select(t=0, s=w427, f=1) -> (s? t:f=w429:i32)
            n254 = property on="Listbox" class="LstBox (strict)"() -> ("Item Symbols"=w432:i32[])  [unwired: 2 in, 2 out]
            n255 = Replace Array Subset(array=w432, new element=w429, index="Listbox") -> (w431:i32[])
            n256 = property on="Listbox" class="LstBox (strict)"("Item Symbols"=w431) -> ()  [unwired: 2 in, 2 out]
          }
          frame Default {
          }
        }
      }
      event "DB Camera Config": Value Change {
        n257 = event-data() -> ("NewVal"=w436:bool)  [unwired: 1 in]
        n258 = case shown="False" w436 {
          tunnel: w435 -> [w445 _]
          tunnel: [w438 w456] -> w434
          tunnel: w433 -> [w437 w456]
          frame False {
            w452 = "Camera"
            w455 = FALSE ("Visible")
            n259 = local read "Camera Settings"() -> (w444:T1)
            n260 = Index Array(array=w445) -> (element=w448:cluster{string[]})  [unwired: 1 in]
            n261 = Unbundle(w444) -> ("Frate Rate"=w443:i32, "Compression"=w442:i32, "Size"=w446:u16)
            n262 = Unbundle(w448) -> (w447:string[])
            n263 = Index Array(array=w447, index=w446) -> (element=w441:string)
            n264 = call-poly <vilib>:"Write Key.vi"("section"=w452, "value"=w441, "key"="Size", "refnum"=w437) -> ("refnum out"=w454:T34)  [unwired: 2 in, 5 out]
            n265 = call-poly <vilib>:"Write Key.vi"("section"=w452, "value"=w443, "key"="FrameRate", "refnum"=w454) -> ("refnum out"=w453:T34)  [unwired: 1 in, 6 out]
            n266 = property on="Camera Settings" class="Clust (strict)"("Visible"=w455) -> ()  [unwired: 2 in, 2 out]
            n267 = local write "DB Camera Config"(w455) -> ()
            n268 = call-poly <vilib>:"Write Key.vi"("section"=w452, "value"=w442, "key"="Compression", "refnum"=w453) -> ("refnum out"=w439:T34)  [unwired: 1 in, 6 out]
            n269 = call <vilib>:"Close Config Data.vi"("refnum"=w439) -> ("file path"=w440:path)  [unwired: 2 in, 8 out]
            n270 = call <vilib>:"Open Config Data.vi"("configuration file path"=w440) -> ("refnum"=w438:T34)  [unwired: 8 in, 2 out]
          }
          frame True {
            n271 = property on="Camera Settings" class="Clust (strict)"("Visible"=TRUE) -> ()  [unwired: 2 in, 2 out]
          }
        }
      }
      event "Camera Settings": Value Change {
        n272 = event-data() -> ("NewVal"=w469:T1)  [unwired: 1 in]
        n273 = Index Array(array=w465) -> (element=w464:cluster{string[]})  [unwired: 1 in]
        n274 = Unbundle(w469) -> ("Frate Rate"=w460:i32, "Compression"=w459:i32, "Size"=w462:u16)
        n275 = Unbundle(w464) -> (w463:string[])
        n276 = Index Array(array=w463, index=w462) -> (element=w461:string)
        n277 = Format Into String(format string="%s   %dfps   %d%%", w461, w460, w459) -> (resulting string=w466:string)  [unwired: 2 in, 1 out]
        n278 = Build Array(w466) -> (w467:string[])
        n279 = property on="DB Camera Config" class="Bool (strict)"("Strings [4]"=w467) -> ()  [unwired: 2 in, 2 out]
      }
      event "Motor.Enable": Value Change {
        n280 = event-data() -> ("NewVal"=w475:bool)  [unwired: 1 in]
        n281 = Unbundle("Motor") -> ("Value"=w474:dbl)  [unwired: 1 out]
        n282 = Select(t=w474, s=w475, f=0.0) -> (s? t:f=w472:dbl)
        n283 = call <vilib>:"NT Write Number.vi"("Numeric"=w472, "Name"=w471) -> ()  [unwired: 9 in, 1 out]
      }
      event "Slider": Value Change {
        n284 = event-data() -> ("NewVal"=w478:dbl)  [unwired: 1 in]
        n285 = call <vilib>:"NT Write Number.vi"("Numeric"=w478, "Name"=w479) -> ()  [unwired: 9 in, 1 out]
      }
      event "On/Off": Value Change {
        n286 = event-data() -> ("NewVal"=w483:bool)  [unwired: 1 in]
        n287 = Boolean To (0,1)(Boolean=w483) -> (0, 1=w482:i16)
        n288 = call <vilib>:"NT Write Number.vi"("Numeric"=w482, "Name"=w481) -> ()  [unwired: 9 in, 1 out]
      }
      event "Rev/Fwd": Value Change {
        n289 = event-data() -> ("NewVal.Forward"=w491:bool, "NewVal.Reverse"=w490:bool)  [unwired: 1 in]
        n290 = Boolean To (0,1)(Boolean=w491) -> (0, 1=w487:i16)
        n291 = Boolean To (0,1)(Boolean=w490) -> (0, 1=w489:i16)
        n292 = Negate(x=w489) -> (-x=w488:i16)
        n293 = Add(x=w487, y=w488) -> (x+y=w486:i16)
        n294 = call <vilib>:"NT Write Number.vi"("Numeric"=w486, "Name"=w485) -> ()  [unwired: 9 in, 1 out]
      }
      event "Ring": Value Change {
        n295 = event-data() -> ("NewVal"=w495:u16)  [unwired: 1 in]
        n296 = property on="Ring" class="Ring (strict)"() -> ("Strings []"=w496:string[])  [unwired: 2 in, 2 out]
        n297 = Index Array(array=w496, index=w495) -> (element=w494:string)
        n298 = call <vilib>:"NT Write String.vi"("String"=w494, "Name"=w493) -> ()  [unwired: 9 in, 1 out]
      }
    }
  }
  n299 = Index Array(array=w20) -> (element=w21:cluster{string[]})  [unwired: 1 in]
  n300 = Unbundle(w21) -> (w19:string[])
  n301 = Match First String(2:w19, 3:w18) -> (0:w17:i32)  [unwired: 1 out]
  n302 = Bundle("value"=w23, "value"=w22, "index"=w17) -> (w11:cluster{"value":i32, "value":i32, "index":i32})  [unwired: 1 out]
  n303 = property on="On/Off" class="Bool (strict)"("Visible"=w34) -> ()  [unwired: 2 in, 2 out]
  n304 = property on="Motor" class="Clust (strict)"("Visible"=w34) -> ()  [unwired: 2 in, 2 out]
  n305 = property on="Progress" class="Clust (strict)"("Visible"=w34) -> ()  [unwired: 2 in, 2 out]
  n306 = property on="Ring" class="Ring (strict)"("Visible"=w34) -> ()  [unwired: 2 in, 2 out]
  n307 = property on="Camera Settings" class="Clust (strict)"("Val(Sgnl)"=w11) -> ()  [unwired: 2 in, 2 out]
  n308 = property on="Rev/Fwd" class="Clust (strict)"("Visible"=w34) -> ()  [unwired: 2 in, 2 out]
  n309 = property on="Camera Settings" class="Clust (strict)"("Visible"=w34) -> ()  [unwired: 2 in, 2 out]
  n310 = local write "DB Camera Config"(w34) -> ()
  n311 = while {
    stop <- FALSE stop-if-true
    # "Shooter Debug Panel"
    # "Front Panel"
    # "Whiteboard:                               y = -2.6332x + 68.073\nTesting 2.23.13                           y = 0.2002x2 - 7.6337x + 101.11\nTesting 2.24.13                           y = 0.2086x2 - 7.5585x + 94.621\nField Test (Orch room) 3.2.13  y = 0.0733x2 - 3.2492x + 59.29\nField Test (Orch room) 3.3.13  y = 0.0782x2 - 3.7527x + 65.268\nLonestar Thursday 3.7.13         y = 0.0872x2 - 3.5994x + 63.288 \nLonestar Friday 3.8.13               y = 0.178x2 - 6.8038x + 91.639\nPrePeachtree 3.11.13                 y = -0.0522x2 + 0.9287x + 27.34"
    n312 = Wait (ms)(milliseconds to wait=u32 60) -> ()  [unwired: 1 out]
    n313 = call "Elapsed Times.vi"("Call Name"="Vision Output") -> ()  [unwired: 2 in, 1 out]
    n314 = local read "Vision/Target Found"() -> (w567:bool)
    n315 = local read "Vision Distance (ft)"() -> (w541:dbl)
    n316 = local read "Shooter/Control/Manual Dist Enabled"() -> (w569:bool)
    n317 = local read "Shooter/Control/Manual Dist"() -> (w570:dbl)
    n318 = Select(t=w541, s=w567, f="Default Distance (ft)") -> (s? t:f=w540:dbl)
    "Camera Distance 2" <- w540
    n319 = call <vilib>:"SD Read Number.vi"("Name"="Azimuth/X Output") -> ("Numeric"=→"Azimuth/X Output 2":dbl)  [unwired: 8 in, 2 out]
    n320 = Select(t=w570, s=w569, f=w540) -> (s? t:f=w536:dbl)
    "Shoot Distance" <- w536
    "Shoot Distance 2" <- w536
    n321 = local read "Elevator Angle Offset"() -> (w539:dbl)
    n322 = Square(x=w536) -> (x^2=w537:dbl)
    n323 = Multiply(x=w537, y="Angle Equation x2") -> (x*y=w532:dbl)
    n324 = Multiply(x=w536, y="Angle Equation x1") -> (x*y=w531:dbl)
    n325 = Compound Arithmetic op=ADD(w532, w531, "Angle Equation x0", w539) -> (w538:dbl)
    n326 = disable-structure shown="Disabled" {
      disable-tunnel: w536 -> [w584 _]
      frame Disabled {
        n327 = expression code="x"(w584) -> (w590:dbl)
        n328 = expression code="x"(w584) -> (w589:dbl)
        n329 = local read "Shooter/Control/Manual Main RPM"() -> (w593:dbl)
        n330 = local read "Shooter/Control/Manual Pre RPM"() -> (w592:dbl)
        n331 = local read "Shooter/Control/Manual RPM"() -> (w591:bool)
        n332 = Select(t=w593, s=w591, f=w590) -> (s? t:f=w586:dbl)
        n333 = Select(t=w592, s=w591, f=w589) -> (s? t:f=w585:dbl)
        n334 = call <vilib>:"SD Write Number.vi"("Numeric"=w585, "Name"="Shooter/Control/Vision Pre RPM") -> ()  [unwired: 8 in, 2 out]
        n335 = call <vilib>:"SD Write Number.vi"("Numeric"=w586, "Name"="Shooter/Control/Vision Main RPM") -> ()  [unwired: 8 in, 2 out]
        n336 = local write "Shooter/Control/Vision Pre RPM"(w585) -> ()
        n337 = local write "Shooter/Control/Vision Main RPM"(w586) -> ()
      }
      frame Enabled {
      }
    }
    n338 = disable-structure shown="Enabled" {
      disable-tunnel: w538 -> [w574 w581]
      frame Disabled {
        n339 = local read "Elevator/Manual Elevation"() -> (w577:dbl)
        n340 = local read "Elevator/Manual Elevation Enabled"() -> (w576:bool)
        n341 = Select(t=w577, s=w576, f=w574) -> (s? t:f=w575:dbl)
        n342 = local write "Elevator/Vision Angle"(w575) -> ()
        n343 = call <vilib>:"SD Write Number.vi"("Numeric"=w575, "Name"="Elevator/Vision Angle") -> ()  [unwired: 8 in, 2 out]
      }
      frame Enabled {
        n344 = Select(t="Manual Angle", s="Manual Elevation Enabled", f=w581) -> (s? t:f=w578:dbl)
        n345 = local read "Shoot Vision"() -> (w580:T4)
        n346 = Bundle By Name(cluster=w580, "Angle"=w578) -> (w579:T4)
        n347 = local write "Shoot Vision"(w579) -> ()
        "Vision Elevation" <- w581
      }
    }
    n348 = call <vilib>:"SD Read String.vi"("Name"="Shoot/Location") -> ("String"=w499:string)  [unwired: 8 in, 2 out]
    n349 = Scan From String(input string=w499, default 1=Shoot_Location."Vision" ("y")) -> (output 1=w497:T36)  [unwired: 3 in, 3 out]
    n350 = Equal?(x=w497, y=Shoot_Location."Front") -> (x = y?=→"Shoot Active Front":bool)
    n351 = Equal?(x=w497, y=Shoot_Location."Front Corner") -> (x = y?=→"Shoot Active Front Corner":bool)
    n352 = Equal?(x=w497, y=Shoot_Location."Back Corner") -> (x = y?=→"Shoot Active Back Corner":bool)
    n353 = Equal?(x=w497, y=Shoot_Location."Half Court") -> (x = y?=→"Shoot Active Half Court":bool)
    n354 = Equal?(x=w497, y=Shoot_Location."Full Court") -> (x = y?=→"Shoot Active Full Court":bool)
    n355 = Equal?(x=w497, y=Shoot_Location."Vision") -> (x = y?=→"Shoot Active Vision":bool)
    n356 = Equal?(x=w497, y=Shoot_Location."Pyramid") -> (x = y?=→"Shoot Active Pyramid":bool)
    n357 = call <vilib>:"SD Read Number.vi"("Name"="Shooter/Control/Target Pre RPM") -> ("Numeric"=→"Shooter/Control/Target Pre RPM":dbl)  [unwired: 8 in, 2 out]
    n358 = call <vilib>:"SD Read Number.vi"("Name"="Elevator/Angle") -> ("Numeric"=→"Elevator/Angle 2" →"Elevator/Angle 3":dbl)  [unwired: 8 in, 2 out]
    n359 = call <vilib>:"SD Read Number.vi"("Name"="Shooter/Control/Target Main RPM") -> ("Numeric"=→"Shooter/Control/Target Main RPM":dbl)  [unwired: 8 in, 2 out]
    n360 = call <vilib>:"SD Read Number.vi"("Name"="Shooter/Output/Pre RPM") -> ("Numeric"=→"Shooter/Output/Pre RPM":dbl)  [unwired: 8 in, 2 out]
    n361 = call <vilib>:"SD Read Number.vi"("Name"="Shooter/Output/Main RPM") -> ("Numeric"=→"Shooter/Output/Main RPM":dbl)  [unwired: 8 in, 2 out]
    n362 = call <vilib>:"SD Read Number.vi"("Name"="Shooter/Output/Pre") -> ("Numeric"=→"Shooter/Output/Pre":dbl)  [unwired: 8 in, 2 out]
    n363 = call <vilib>:"SD Read Number.vi"("Name"="Shooter/Output/Main") -> ("Numeric"=→"Shooter/Output/Main":dbl)  [unwired: 8 in, 2 out]
    n364 = call <vilib>:"SD Read Number.vi"("Name"="Elevator/Output/Target Angle") -> ("Numeric"=→"Elevator/Output/Target Angle 2" →"Elevator/Output/Target Angle 3":dbl)  [unwired: 8 in, 2 out]
    n365 = call <vilib>:"SD Read Number.vi"("Name"="Sensor/Shooter Pot/Value") -> ("Numeric"=→"Sensor/Shooter Pot/Value":dbl)  [unwired: 8 in, 2 out]
    n366 = call <vilib>:"SD Read Boolean.vi"("Name"="Shooter/Output/RPM Ready") -> ("Boolean"=→"Shooter/Output/RPM Ready 2":bool)  [unwired: 8 in, 2 out]
    n367 = call <vilib>:"SD Read Boolean.vi"("Name"="Elevator/Output/Shoot Angle Ready") -> ("Boolean"=→"Elevator/Output/Shoot Angle Ready 2":bool)  [unwired: 8 in, 2 out]
    n368 = call <vilib>:"SD Read Boolean.vi"("Name"="Shooter/Output/Azimuth Ready") -> ("Boolean"=→"Shooter/Output/Azimuth Ready 2":bool)  [unwired: 8 in, 2 out]
    n369 = call <vilib>:"SD Read Boolean.vi"("Name"="Shooter/Output/Shooter Ready") -> ("Boolean"=→"Shooter/Output/Shooter Ready 2":bool)  [unwired: 8 in, 2 out]
    n370 = call <vilib>:"SD Read Boolean.vi"("Name"="Shooter/Output/Flipper Output") -> ("Boolean"=→"Shooter/Output/Flipper Output 2":bool)  [unwired: 8 in, 2 out]
    n371 = call <vilib>:"SD Read Boolean.vi"("Name"="Auto/Load Ramp Down") -> ("Boolean"=w547:bool)  [unwired: 8 in, 2 out]
    "Auto/Load Ramp Down" <- w547
    n372 = call <vilib>:"SD Read Number.vi"("Name"="Drive/Gear") -> ("Numeric"=→"Drive Gear":dbl)  [unwired: 8 in, 2 out]
    n373 = call <vilib>:"SD Read Number.vi"("Name"="Sensor/Gyro/Angle") -> ("Numeric"=→"Gyro Angle":dbl)  [unwired: 8 in, 2 out]
    n374 = call <vilib>:"SD Read Boolean.vi"("Name"="Azimuth/Auto Enabled") -> ("Boolean"=→"Azmuth Enabled":bool)  [unwired: 8 in, 2 out]
    n375 = call <vilib>:"SD Read Boolean.vi"("Name"="Elevator/Auto Enabled") -> ("Boolean"=→"Elevator Enabled":bool)  [unwired: 8 in, 2 out]
    n376 = property on="Auto/Load Ramp Down" class="Bool (strict)"("Blinking"=w547) -> ()  [unwired: 2 in, 2 out]
  }
  n377 = String To IP(1:"10.06.24.02" ("name")) -> (0:w3:u32)
  n378 = UDP Open(11:w2) -> (port=w4:refnum<k16>)  [unwired: 4 in, 2 out]
  n379 = while {
    tunnel: w3 -> [w642]
    tunnel: w2 -> [w641]
    tunnel: T20 {"Feed Angle"=20.0, "Neutral Angle"=25.8, "Autonomous Setpoints"={"Shoot Angle 1"=3500.0, "Initial Delay"=4000.0, "Disc Count 1"=27.0, "Shoot Time 1"=0.0, "Distance 1"=0.0, "Two Disc Distance 1"=0.0, "Distance 2"=0.0, "Two Disc Distance 2"=0.0, "Distance 3"=0.0, "Two Disc Distance 3"=0.0, "Shoot Angle 3"=0.0, "Disc Count 3"=0.0, "Shoot Time 3"=0.0, "Distance 4"=0.0, "Two Disc Distance 4"=0.0, "Low Gear"=FALSE, "Shoot 1 Post Delay"=0.0}, "Auto Shift"={"Enabled"=FALSE, "Upshift Speed"=4000.0, "Downshift Speed"=27.0, "Upshift Throttle"=0.0, "Turn Power Diff"=0.0, "Motor Limit"=0.0, "Encoder Limit"=0.0}, "Elevator Angle Offset"=0.0, "Potentiometer Angle"={"Pot M"=0.0, "Pot B"=0.0}, "Shoot Setpoints"={"Vision"={"Pre RPM"=0.0, "Main RPM"=0.0, "Angle"=0.0}, "Back Corner"={"Pre RPM"=0.0, "Main RPM"=0.0, "Angle"=0.0}, "Front"={"Pre RPM"=0.0, "Main RPM"=0.0, "Angle"=0.0}, "Front Corner"={"Pre RPM"=0.0, "Main RPM"=0.0, "Angle"=0.0}, "Half Court"={"Pre RPM"=0.0, "Main RPM"=0.0, "Angle"=0.0}, "Full Court"={"Pre RPM"=0.0, "Main RPM"=0.0, "Angle"=0.0}, "Pyramid"={"Pre RPM"=0.0, "Main RPM"=0.0, "Angle"=0.0}}, "Halo Drive"={"Gains"={"Quickturn_Sens_Low"=0.0, "Quickturn_Sens_High"=0.0, "Speedturn_Sens_Low"=0.0, "Speedturn_Sens_High"=0.0}, "QuickTurn Const"=0.0, "Loading Throttle Limit"=0.0}, "Auto Speed Constants"={"Slowing Distance"=0.0, "High Speed"=0.0, "Rampup Time"=0.0, "Low Speed"=0.0, "High Speed (Reverse)"=0.0}, "Shooting Delays"={"Unjam On"=0.0, "Unjam Off"=0.0, "Flipper On"=0.0, "Flipper Off"=0.0, "Hopper Up"=0.0}, "Left Roller Pwr"=0.0, "Right Roller Pwr"=0.0, "Elevator PID Gains"={"proportional gain (Kc)"=0.0, "integral time (Ti, min)"=0.0, "derivative time (Td, min)"=0.0}, "Elevator PID Output Range"={"output high"=0.0, "output low"=0.0}, "Elevator Angle Tolerance"=0.0, "Toggle Ears Delay"=0.0, "Toggle Ears Distance"=0.0, "Unjam Servo Angle"=0.0, "Auton Steer PID gains"={"proportional gain (Kc)"=0.0, "integral time (Ti, min)"=0.0, "derivative time (Td, min)"=0.0}, "Auton Steer output range"={"output high"=0.0, "output low"=0.0}, "Auto Reverse Speed"=0.0, "Auto Stop Throttle"=0.0, "Auto Stop Duration"=0.0, "Spin output range"={"output high"=0.0, "output low"=0.0}, "Spin PID gains"={"proportional gain (Kc)"=0.0, "integral time (Ti, min)"=0.0, "derivative time (Td, min)"=0.0}, "Auto-Center Line"={"Arc Turn x-axis"=0.0, "Arc Turn y-axis"=0.0, "Arc Turn Distance"=0.0, "Distance 1"=0.0, "Two Disc Distance 1"=0.0, "Distance 2"=0.0, "Two Disc Distance 2"=0.0, "Spin Angle"=0.0, "Spin Angle tolerance"=0.0, "Spin y-axis"=0.0, "Spin Distance"=0.0, "Center Line Enabled"=FALSE, "Distance 3"=0.0, "Two Disc Distance 3"=0.0, "Spin Angle 2"=0.0, "Spin Angle tolerance 2"=0.0, "Spin y-axis 2"=0.0, "Spin Distance 2"=0.0, "Shoot Angle 1"=0.0, "Disc Count 1"=0.0, "Shoot Time 1"=0.0, "Shoot Angle 3"=0.0, "Disc Count 3"=0.0, "Shoot Time 3"=0.0, "Low Gear"=FALSE}, "Auton Distance PID gains Low Gear"={"proportional gain (Kc)"=0.0, "integral time (Ti, min)"=0.0, "derivative time (Td, min)"=0.0}, "Auton Distance output range"={"output high"=0.0, "output low"=0.0}, "Auton Distance Threshold"=0.0, "Auton Velocity Cutoff"=0.0, "Auton Distance output range Center Line"={"output high"=0.0, "output low"=0.0}, "Auton Distance PID gains High Gear"={"proportional gain (Kc)"=0.0, "integral time (Ti, min)"=0.0, "derivative time (Td, min)"=0.0}} ("UDP Packet") -> [w640]
    shift-right: [w638] -> _
    shift-left: w4 -> [w643]
    stop <- FALSE stop-if-true
    n380 = Bundle By Name(cluster=T37 {"Vision"={"Pre RPM"=3500.0, "Main RPM"=4000.0, "Angle"=16.4}, "Back Corner"={"Pre RPM"=3500.0, "Main RPM"=4000.0, "Angle"=16.3}, "Front"={"Pre RPM"=3500.0, "Main RPM"=4000.0, "Angle"=23.5}, "Front Corner"={"Pre RPM"=3500.0, "Main RPM"=4000.0, "Angle"=21.8}, "Half Court"={"Pre RPM"=3500.0, "Main RPM"=4000.0, "Angle"=16.4}, "Full Court"={"Pre RPM"=4500.0, "Main RPM"=5000.0, "Angle"=16.0}, "Pyramid"={"Pre RPM"=2800.0, "Main RPM"=3300.0, "Angle"=28.0}} ("Shoot Setpoints"), "Vision"="Shoot Vision", "Front"="Shoot Front", "Back Corner"="Shoot Back Corner", "Front Corner"="Shoot Front Corner", "Half Court"="Shoot Half Court", "Full Court"="Shoot Full Court", "Pyramid"="Shoot Pyramid") -> (w631:T37)
    n381 = Bundle By Name(cluster=w640, "Feed Angle"="Feed Angle", "Neutral Angle"="Neutral Angle", "Autonomous Setpoints"="Autonomous Setpoints", "Auto Shift"="Auto Shift", "Elevator Angle Offset"="Elevator Angle Offset", "Potentiometer Angle"="Potentiometer Angle", "Shoot Setpoints"=w631, "Halo Drive"="Halo Drive", "Toggle Ears Delay"="Toggle Ears Delay", "Auto Speed Constants"="Auto Speed Constants", "Shooting Delays"="Shooting Delays", "Left Roller Pwr"="Left Roller Pwr", "Right Roller Pwr"="Right Roller Pwr", "Elevator PID Gains"="Elevator PID Gains", "Elevator PID Output Range"="Elevator PID Output Range", "Elevator Angle Tolerance"="Angle Tolerance", "Toggle Ears Distance"="Toggle Ears Distance", "Unjam Servo Angle"="Unjam Servo Angle", "Auton Steer PID gains"="Auton Steer PID gains", "Auton Steer output range"="Auton Steer output range", "Auto Reverse Speed"="Auto Reverse Speed", "Auto Stop Throttle"="Auto Stop Throttle", "Auto Stop Duration"="Auto Stop Duration (ms)", "Spin output range"="Auton Spin output range", "Spin PID gains"="Auton Spin PID gains", "Auto-Center Line"="Auto-Center Line", "Auton Distance PID gains Low Gear"="Auton Distance PID gains\nLow Gear", "Auton Distance output range"="Auton Distance output range", "Auton Distance Threshold"="Auton Distance Threshold", "Auton Velocity Cutoff"="Auton Velocity Cutoff", "Auton Distance output range Center Line"="Auton Distance output range\nCenter Line", "Auton Distance PID gains High Gear"="Auton Distance PID gains\nHigh Gear") -> (w611:T20)
    n382 = Flatten To String(anything=w611) -> (data string=w604:string)  [unwired: 3 in, 2 out]
    n383 = UDP Write(address=w642, port or service name=w641, connection ID=w643, data in=w604) -> (3:w638:refnum<k16>)  [unwired: 2 in, 1 out]
    n384 = String Length(string=w604) -> (length=→"UDP packet length":i32)
    n385 = Wait (ms)(milliseconds to wait=u32 100) -> ()  [unwired: 1 out]
  }
